vi "MP-Message Decoder.vi"(8 "error in (no error)":errorcluster, 10 "SDO messages":string="#y\u0010\u0000\u0007\u0007\u0001dd\u0001$\u0007\u0007\u0003\u0018ÿ\u0018\u0018\u0018\u0018\u0018\u0018\u0018\u0018)\u0000\u0007\u0007\u0001\u001a", 11 "data controls":T1={"Scan Reset"=FALSE, "Sub Sampling"=1, "Report Data Msg"=FALSE} {"Sub Sampling" items=["", "1:1", "2:1", "3:1", "4:1", "5:1", "6:1", "7:1", "8:1", "9:1", "10:1"]}) -> (0 "error out":errorcluster, 1 "System Status":T5={"System Type"=enum."MicroPulse 5", "Serial No."=0, "Channels"={"Conv"=0, "PA"=0, "Extra"=0}, "Sample Frequency"={"Default"=0, "Actual"=0}, "Software Versions"="", "Data Output Format"={"Default"=enum."8-bit Mode", "Actual"=enum."8-bit Mode"}, "Temperatures"={"System"=0, "Processor"=0, "Slave Sys"=0, "Slave Proc"=0}, "Tx Buffer Size"=0, "System Error"="", "No. of Cards"=0, "DAC Gain"=0, "Uptimes"={"since Power"=0, "since RSTS"=0, "since SRST"=0}, "Voltages"=[], "Interface Cards"=[]} {"Interface Cards"."FPGA - T" format="%.0f °C"; "Interface Cards"."Board - T" format="%.0f °C"; "Voltages"."Difference" format="%.2fV"; "Voltages"."Measured" format="%.2fV"; "Voltages"."Nominal" format="%.2fV"; "DAC Gain" format="%.0fdB"; "Tx Buffer Size" format="%.0fMB"; "Temperatures"."Slave Proc" format="%.0f C"; "Temperatures"."Slave Sys" format="%.0f C"; "Temperatures"."Processor" format="%.0f C"; "Temperatures"."System" format="%.0f C"; "Sample Frequency"."Actual" format="%.0fMHz"; "Sample Frequency"."Default" format="%.0fMHz"}, 2 "scan data info":T9={"Message Header"=0, "Error Message"=0, "Test No."=0, "Channel No."=0, "Sweep No."=0, "Gate No."=0, "DOF"=enum."8-bit Mode", "retain data"=enum."Ascan", "scan data"=[], "scan length"=0, "scan index"=0, "peak data"={"timebase"=[], "data"=[]}, "#peaks"=0, "PRF"=0.0, "IP"={"Axis No."=0, "Location"=0, "MIP location"=0, "MIP?"=FALSE}, "echo range"=0, "ETG"=FALSE, "CAL 0 complete"=FALSE, "Axis Positions"={"Axis 1"=0, "Axis 2"=0, "Axis 3"=0, "Axis 4"=0, "Status"=0}} {"Error Message" format="%04x"; "Message Header" format="%04x"; "IP"."MIP location" format="%#.0f"; "IP"."Location" format="%#.0f"; "PRF" format="%.0fHz"}, 3 "Instrument Message":string="A-Scan\n---------\n\rLength = 108 bytes\nSweep No. 0\nTest No. 0\nDOF = MicroPulse 4\nerror\nChannel No. 0", 4 "reported msg length":u32 format="%d bytes", 5 "Axis Status":T3 {"IO Levels"."Outputs: 7-0" format="%.0b"; "IO Levels"."Outputs: 15-8" format="%.0b"; "IO Levels"."Inputs: 7-0" format="%.0b"; "IO Levels"."Inputs: 15-8" format="%.0b"}, 7 "message header":u16 format="%04x")   [LabVIEW 2026, in "MicroPulse_Driver.lvlib"]
doc: "MicroPulse standard data output message decoder.\n\nNote:\n\n1. Currently only supports LT/LT2 instruments.\n2. Supports LT/LT2/MP5\n3. Supports LTPA.\n\n\nDeon Bester\n2018/11/10"
uses:
  MicroPulse_Driver.lvlib
  Datatypes/MP - scan data info.ctl
  Datatypes/MP - data output format.ctl
  Datatypes/MP - retain scan.ctl
  Datatypes/MP - axis positions (LLC).ctl
  Datatypes/MP - general system status.ctl
  <instrlib>/MicroPulse/Public/Data/Datatypes/MP - instrument type.ctl
  Datatypes/MP - interface card status.ctl
  Datatypes/MP - axis status.ctl
  Datatypes/MP - extracted data controls.ctl
  Datatypes/PNDT - subsampling.ctl
  <vilib>/ptbypt/NI_PtbyPt.lvlib
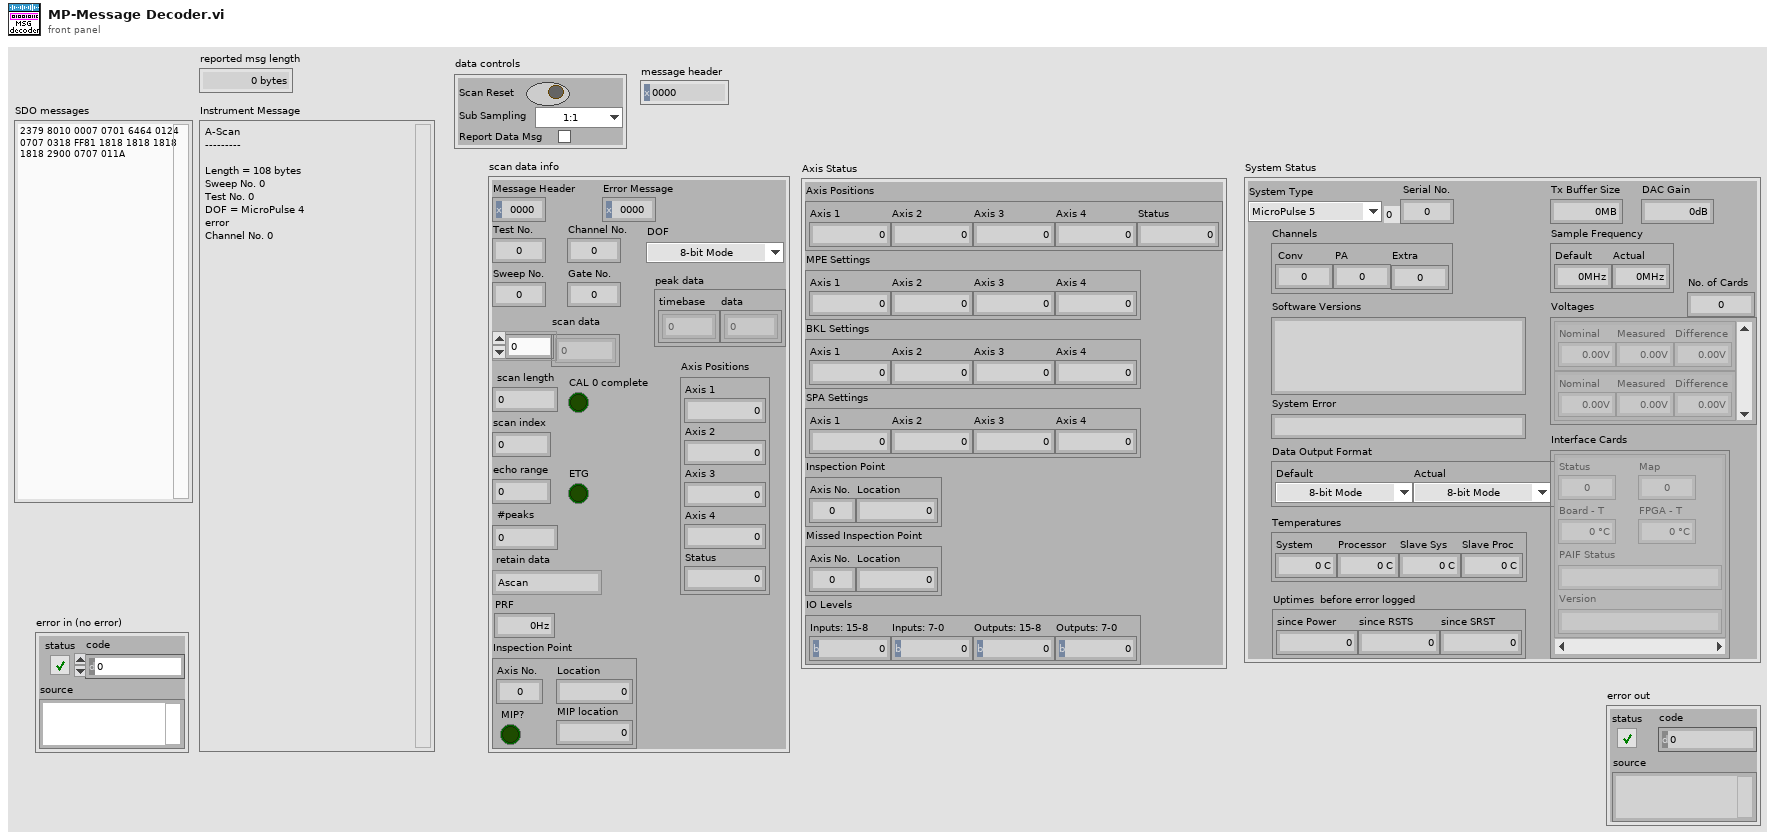
[diagram p1: front panel]
types:
  T1 = typedef "MicroPulse_Driver.lvlib/MP - extracted data controls.ctl" = cluster{"Scan Reset":bool, "Sub Sampling":T2, "Report Data Msg":bool}
  T2 = typedef "MicroPulse_Driver.lvlib/PNDT - subsampling.ctl" = u16
  T3 = typedef "MicroPulse_Driver.lvlib/MP - axis status.ctl" = cluster{"Axis Positions":T4, "MPE Settings":cluster{"Axis 1":u32, "Axis 2":u32, "Axis 3":u32, "Axis 4":u32}, "BKL Settings":cluster{"Axis 1":u32, "Axis 2":u32, "Axis 3":u32, "Axis 4":u32}, "SPA Settings":cluster{"Axis 1":u32, "Axis 2":u32, "Axis 3":u32, "Axis 4":u32}, "IP":cluster{"Axis No.":u8, "Location":u32}, "MIP":cluster{"Axis No.":u8, "Location":u32}, "IO Levels":cluster{"Inputs: 15-8":u8, "Inputs: 7-0":u8, "Outputs: 15-8":u8, "Outputs: 7-0":u8}}
  T4 = typedef "MicroPulse_Driver.lvlib/MP - axis positions (LLC).ctl" = cluster{"Axis 1":u32, "Axis 2":u32, "Axis 3":u32, "Axis 4":u32, "Status":u8}
  T5 = typedef "MicroPulse_Driver.lvlib/MP - general system status.ctl" = cluster{"System Type":T6, "Serial No.":u64, "Channels":cluster{"Conv":u8, "PA":u16, "Extra":u32}, "Sample Frequency":cluster{"Default":u8, "Actual":u8}, "Software Versions":string, "Data Output Format":cluster{"Default":T7, "Actual":T7}, "Temperatures":cluster{"System":u8, "Processor":u8, "Slave Sys":u8, "Slave Proc":u8}, "Tx Buffer Size":u32, "System Error":string, "No. of Cards":u8, "DAC Gain":i16, "Uptimes":cluster{"since Power":u32, "since RSTS":u32, "since SRST":u32}, "Voltages":cluster{"Nominal":dbl, "Measured":dbl, "Difference":dbl}[], "Interface Cards":T8[]}
  T6 = typedef "MicroPulse_Driver.lvlib/MP - instrument type.ctl" = enum16{"MicroPulse 5", "LT1", "LT2", "LTPA", "MPLT", "MicroPulse 6", "PipeScanner", "<MicroPulse>", "Micropulse 4", "Simulated Data"}
  T7 = typedef "MicroPulse_Driver.lvlib/MP - data output format.ctl" = enum16{"", "8-bit Mode", "10-bit Mode", "12-bit Mode", "16-bit Mode", "8-bit Log Mode", "12-bit Packed Mode"}
  T8 = typedef "MicroPulse_Driver.lvlib/MP - interface card status.ctl" = cluster{"Status":u8, "Map":u8, "Board - T":u8, "FPGA - T":u8, "PAIF Status":string, "Version":string}
  T9 = typedef "MicroPulse_Driver.lvlib/MP - scan data info.ctl" = cluster{"Message Header":u16, "Error Message":u16, "Test No.":u32, "Channel No.":u8, "Sweep No.":u32, "Gate No.":u32, "DOF":T7, "retain data":T10, "scan data":u16[], "scan length":i32, "scan index":i32, "peak data":cluster{"timebase":u16[], "data":u16[]}, "#peaks":i32, "PRF":dbl, "IP":cluster{"Axis No.":u8, "Location":u32, "MIP location":u32, "MIP?":bool}, "echo range":u16, "ETG":bool, "CAL 0 complete":bool, "Axis Positions":T4}
  T10 = typedef "MicroPulse_Driver.lvlib/MP - retain scan.ctl" = enum16{"None", "Ascan", "Peaks"}
  T11 = cluster{"Nominal":dbl, "Measured":dbl, "Difference":dbl}[]
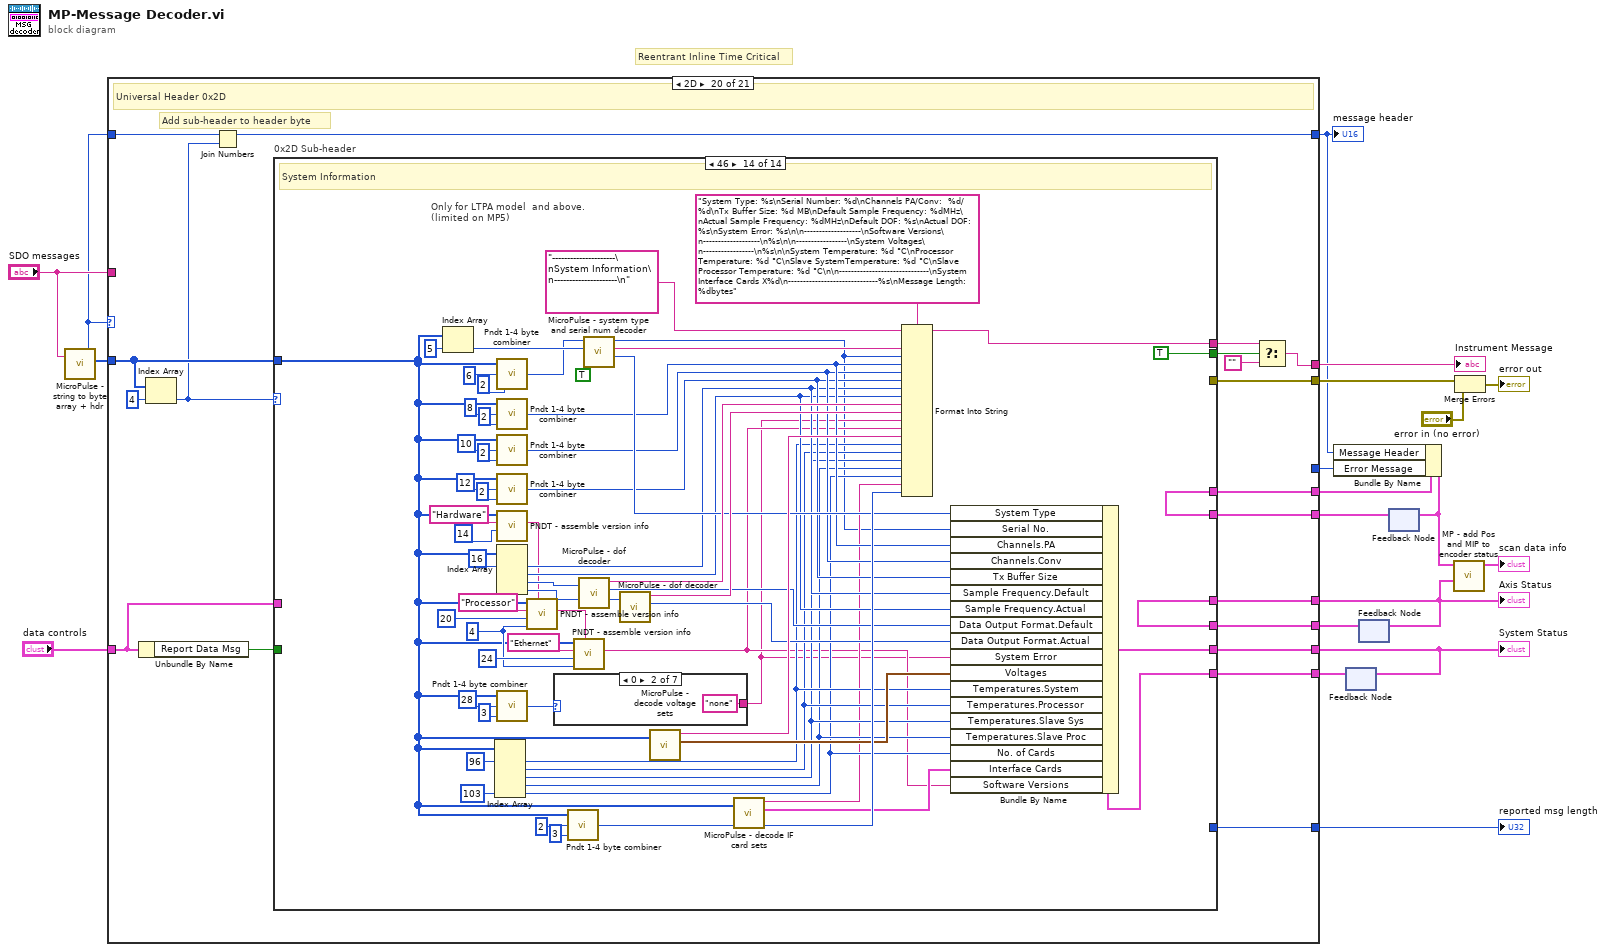
[diagram p0: block diagram]
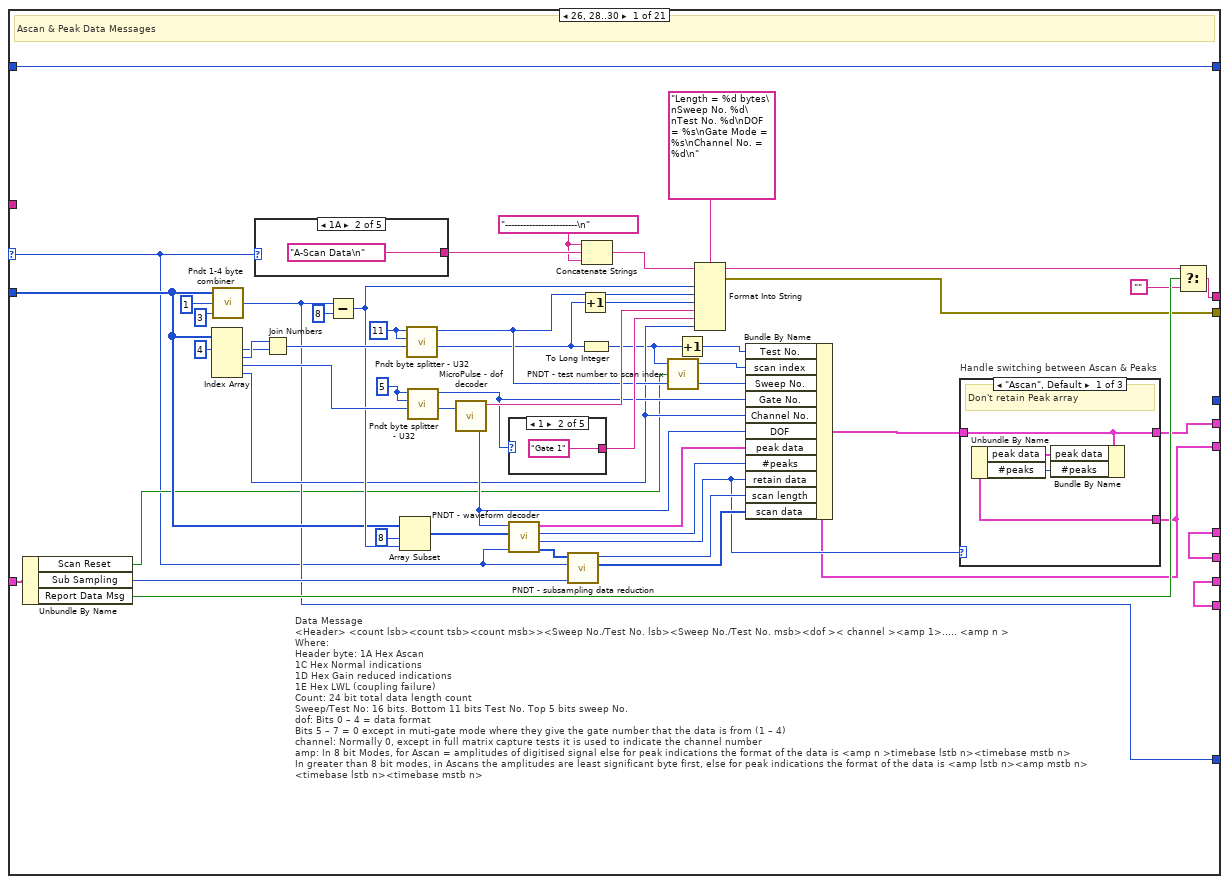
[diagram p2: hidden frame]
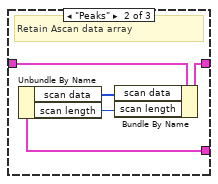
[diagram p3: hidden frame]
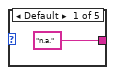
[diagram p5: hidden frame]
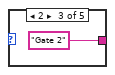
[diagram p6: hidden frame]
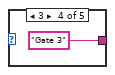
[diagram p7: hidden frame]
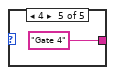
[diagram p8: hidden frame]
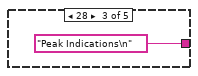
[diagram p10: hidden frame]
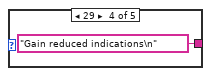
[diagram p11: hidden frame]
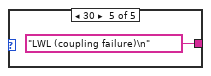
[diagram p12: hidden frame]
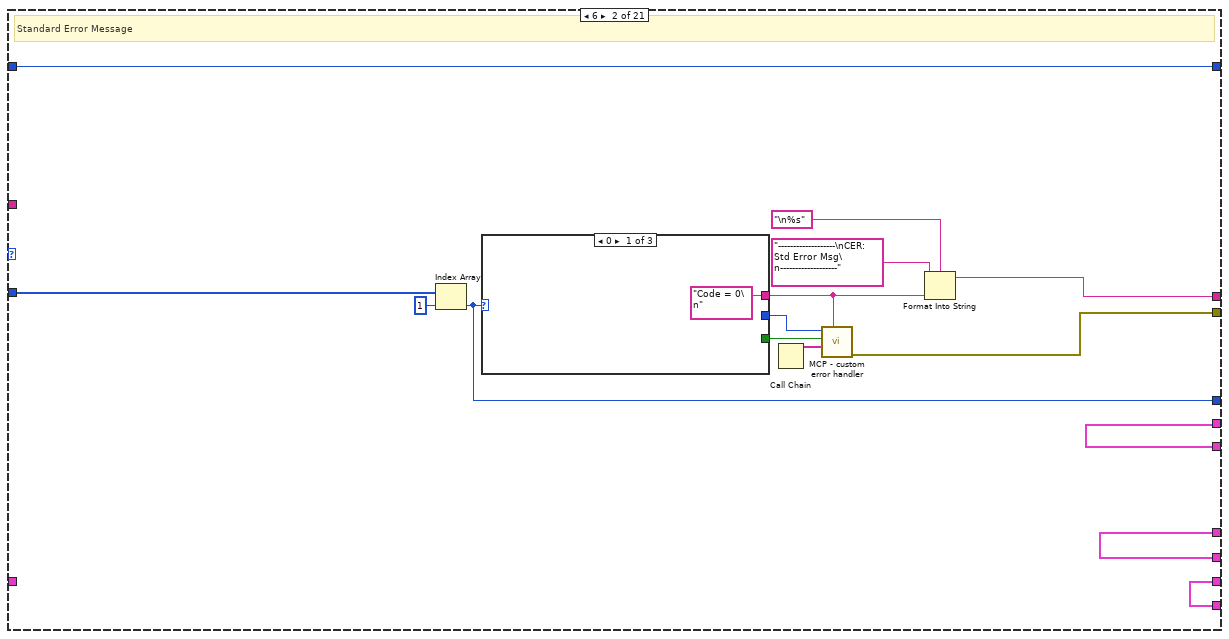
[diagram p13: hidden frame]
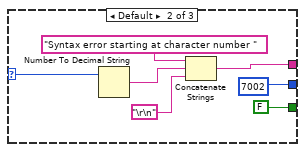
[diagram p14: hidden frame]
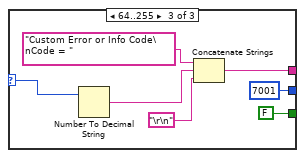
[diagram p15: hidden frame]
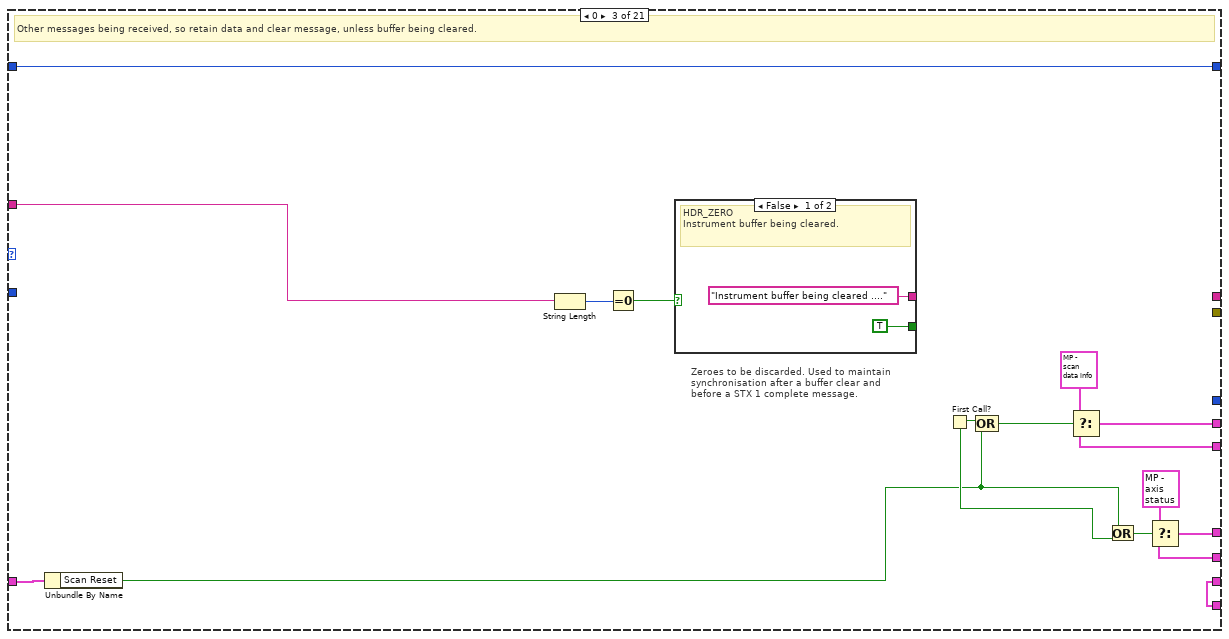
[diagram p16: hidden frame]
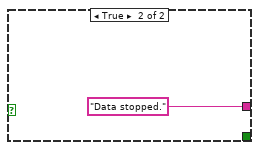
[diagram p17: hidden frame]
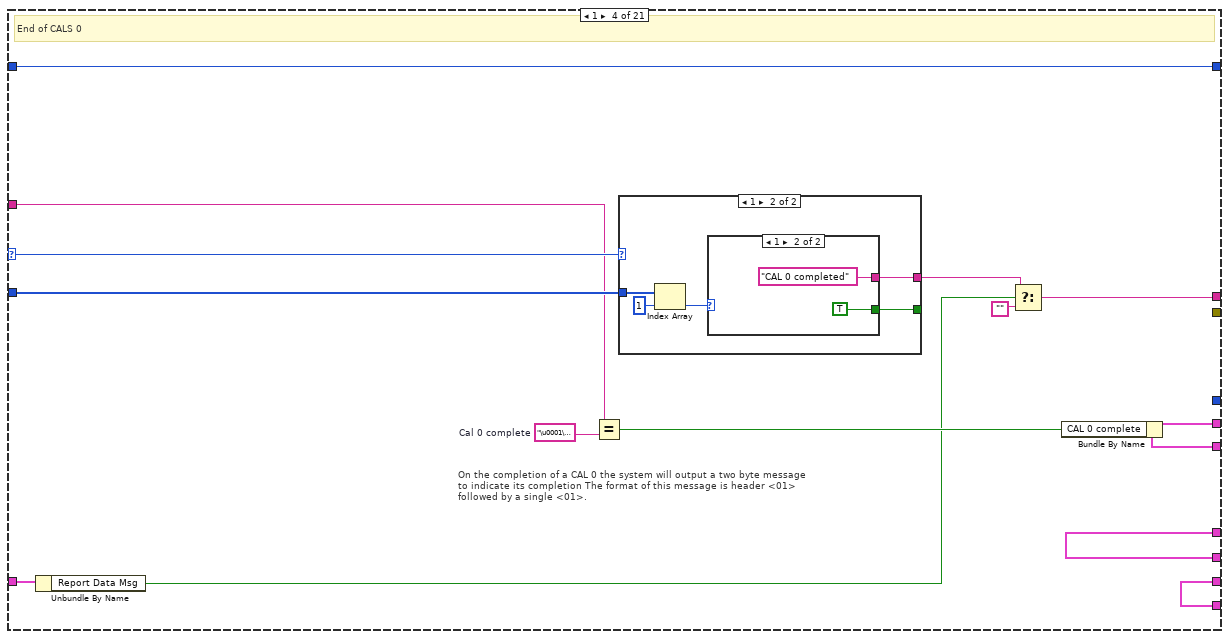
[diagram p18: hidden frame]
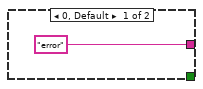
[diagram p19: hidden frame]
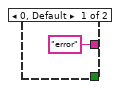
[diagram p20: hidden frame]
diagram:
  # "Reentrant Inline Time Critical"
  n1 = call "MicroPulse - string to byte array + hdr.vi"("SDO msg (hex)"="SDO messages") -> ("header"=w5:u8, "[U8]"=w19:u8[])  [unwired: 3 in]
  n2 = feedback #1() -> (w18:T5)  [unwired: 1 in]
  n3 = feedback #2() -> (w17:T3)  [unwired: 1 in]
  n4 = feedback #3() -> (w14:T9)  [unwired: 1 in]
  n5 = case shown="2D" w5 {
    selector: w5 -> [w24 _ _ w148 _ _ _ _ _ _ _ _ _ _ _ _ _ _ _ _ w1377]
    tunnel: w19 -> [w33 w105 _ w154 w173 w188 w214 w232 w456 w482 w524 w603 w652 w689 w725 w752 w780 w800 w816 w849 _]
    tunnel: [w34 w104 _ w151 w170 w181 w213 w230 w457 w488 w529 w621 w659 w696 w732 w746 w786 w803 w824 w841 w1379] -> w7
    tunnel: w18 -> [w20 w91 w136 w140 w164 w186 w211 w233 w382 w466 w502 _ w631 w668 w705 w741 w770 w790 w807 w847 w1375]
    tunnel: [w28 w99 w129 w152 w166 w175 w210 w231 w384 w468 w504 w574 w633 w670 w707 w748 w772 w792 w809 w845 w1384] -> w16
    tunnel: w17 -> [w28 w99 w130 w152 w166 w187 w212 w235 w384 w468 w504 w574 w633 w670 w707 w748 w772 w792 w809 w846 w1384]
    tunnel: "SDO messages" -> [_ _ w126 w145 _ _ _ _ _ _ _ _ _ _ _ _ _ _ _ _ _]
    tunnel: [w32 w98 _ _ _ _ _ _ _ _ _ _ _ _ _ w751 _ _ _ w844 w1382] -> w6
    tunnel: "data controls" -> [w31 _ w131 w147 _ w180 _ _ _ _ _ _ _ _ _ w745 _ _ _ w838 _]
    tunnel: [w26 w100 w132 w149 w167 w184 w208 w228 w385 w469 w505 w576 w634 w671 w708 w750 w773 w793 w810 w836 w1385] -> w9
    tunnel: w14 -> [w25 w100 w133 w153 w167 w184 w208 w228 w385 w469 w505 w576 w634 w671 w708 w749 w773 w793 w810 w835 w1385]
    tunnel: [w30 _ _ _ _ _ _ _ _ _ _ _ _ _ _ _ _ _ _ w837 _] -> w12
    tunnel: [w21 w93 w121 w141 w165 w179 w206 w227 w383 w467 w503 w573 w632 w669 w706 w743 w771 w791 w808 w833 w1376] -> w3
    tunnel: w5 -> [w21 w93 w121 w141 w165 w179 w206 w227 w383 w467 w503 w573 w632 w669 w706 w743 w771 w791 w808 w834 w1376]
    tunnel: [_ w92 _ _ _ _ _ _ _ _ _ _ _ _ _ _ _ _ _ _ _] -> w2
    tunnel: [w20 w91 w136 w140 w164 w186 w211 w234 w382 w466 w502 w578 w631 w668 w705 w741 w770 w790 w807 w848 w1375] -> w1
    frame 26, 28..30 {
      w64 = i16 11 ("y")
      w66 = i16 5 ("y")
      w49 = "------------------------\n" ("input 1")
      # "Data Message\n<Header> <count lsb><count tsb><count msb>><Sweep No./Test No. lsb><Sweep No./Test No. msb><dof >< channel ><amp 1>….. <amp n >\nWhere:\nHeader byte: 1A Hex Ascan\n1C Hex Normal indications\n1D Hex Gain reduced indications\n1E Hex LWL (coupling failure)\nCount: 24 bit total data length count\nSweep/Test No: 16 bits. Bottom 11 bits Test No. Top 5 bits sweep No.\ndof: Bits 0 – 4 = data format\nBits 5 – 7 = 0 except in muti-gate mode where they give the gate number that the data is from (1 – 4)\nchannel: Normally 0, except in full matrix capture tests it is used to indicate the channel number\namp: In 8 bit Modes, for Ascan = amplitudes of digitised signal else for peak indications the format of the data is <amp n >timebase lstb n><timebase mstb n>\nIn greater than 8 bit modes, in Ascans the amplitudes are least significant byte first, else for peak indications the format of the data is <amp lstb n><amp mstb n> <timebase lstb n><timebase mstb n>"
      # "Ascan & Peak Data Messages"
      n6 = Unbundle By Name(w31) -> ("Scan Reset"=w29:bool, "Sub Sampling"=w46:T2, "Report Data Msg"=w41:bool)
      n7 = Index Array(array=w33, index #1=4 ("index")) -> (element #1=w57:u8, element #2=w58:u8, element #3=w65:u8, element #4=w51:u8)  [unwired: 3 in]
      n8 = call "Pndt 1-4 byte combiner.vi"("#bytes"=3 ("index"), "start index [0]"=1 ("index"), "[U8] count bytes"=w33) -> ("U32"=w30:u32)
      n9 = case shown="1A" w24 {
        tunnel: [_ "A-Scan Data\n" "Peak Indications\n" "Gain reduced indications\n" "LWL (coupling failure)\n"] -> w69
        frame 0, Default {
        }
        frame 26 {
        }
        frame 28 {
        }
        frame 29 {
        }
        frame 30 {
        }
      }
      n10 = Join Numbers(hi=w58, lo=w57) -> ((hi.lo)=w63:u16)
      n11 = Subtract(x=w30, y=u32 8) -> (x-y=w52:u32)
      n12 = Array Subset "Array Subset"(array=w33, index=8, length=w52) -> (w45:u8[])
      n13 = call "Pndt byte splitter - U32.vi"("byte U32"=w63, "mask size"=w64, "shift right"=w64) -> ("lo"=w44:u32, "hi"=w53:u32)  [unwired: 7 in]
      n14 = call "Pndt byte splitter - U32.vi"("byte U32"=w65, "mask size"=w66, "shift right"=w66) -> ("lo"=w61:u32, "hi"=w54:u32)  [unwired: 7 in]
      n15 = call "MicroPulse - dof decoder.vi"("dof"=w61) -> ("String"=w68:string, "DOF"=w55:T7)  [unwired: 3 in]
      n16 = case shown="1" w54 {
        tunnel: ["n.a." "Gate 1" "Gate 2" "Gate 3" "Gate 4"] -> w67
        frame Default {
        }
        frame 1 {
        }
        frame 2 {
        }
        frame 3 {
        }
        frame 4 {
        }
      }
      n17 = call "PNDT - waveform decoder.vi"("header (1A)"=w24, "[U8]"=w45, "DOF"=w55) -> ("scan data"=w48:u16[], "retain data"=w35:T10, "#peaks"=w38:i32, "XY data"=w39:cluster{u16[], u16[]})  [unwired: 5 in]
      n18 = call "PNDT - subsampling data reduction.vi"("sub-sampling"=w46, "header (1A)"=w24, "data set"=w48) -> ("reduced data set"=w40:u16[], "scan length"=w37:i32)  [unwired: 7 in]
      n19 = Increment(x=w44) -> (x+1=w36:u32)
      n20 = To Long Integer(number=w44) -> (32bit integer=w43:i32)
      n21 = Concatenate Strings(w49, w69, w49) -> (w50:string)
      n22 = call "PNDT - test number to scan index.vi"("reset"=w29, "test no."=w43) -> ("scan index"=w42:i32)  [unwired: 2 in, 1 out]
      n23 = Increment(x=w43) -> (x+1=w22:i32)
      n24 = Format Into String(format string="Length = %d bytes\nSweep No. %d\nTest No. %d\nDOF = %s\nGate Mode = %s\nChannel No. = %d\n", initial string=w50, w52, w53, w36, w68, w67, w51) -> (resulting string=w47:string, error out=w32:errorcluster)  [unwired: 1 in]
      n25 = Bundle By Name(cluster=w25, "Test No."=w22, "scan index"=w42, "Sweep No."=w53, "Gate No."=w54, "Channel No."=w51, "DOF"=w55, "peak data"=w39, "#peaks"=w38, "retain data"=w35, "scan length"=w37, "scan data"=w40) -> (w27:T9)
      n26 = case "Handle switching between Ascan & Peaks" shown="\"Ascan\", Default" w35 {
        tunnel: w27 -> [w72 w79 w81]
        tunnel: [w72 w78 w81] -> w26
        tunnel: w25 -> [w74 w77 _]
        frame "Ascan", Default {
          # "Don't retain Peak array"
          n27 = Unbundle By Name(w74) -> ("peak data"=w75:cluster{"timebase":u16[], "data":u16[]}, "#peaks"=w73:i32)
          n28 = Bundle By Name(cluster=w72, "peak data"=w75, "#peaks"=w73) -> ()  [unwired: 1 out]
        }
        frame "Peaks" {
          # "Retain Ascan data array"
          n29 = Unbundle By Name(w77) -> ("scan data"=w80:u16[], "scan length"=w76:i32)
          n30 = Bundle By Name(cluster=w79, "scan data"=w80, "scan length"=w76) -> (w78:T9)
        }
        frame "None" {
        }
      }
      n31 = Select(t=w47, s=w41, f="") -> (s? t:f=w34:string)
    }
    frame 6 {
      # "Standard Error Message"
      n32 = Index Array(array=w105, index=1) -> (element=w92:u8)
      n33 = case shown="0" w92 {
        selector: w92 -> [_ w113 w115]
        tunnel: ["Code = 0\n" w110 w117] -> w95
        tunnel: [_ 7002 ("custom error code") 7001 ("custom error code")] -> w97
        tunnel: [_ FALSE FALSE] -> w94
        frame 0 {
        }
        frame Default {
          n34 = Number To Decimal String(number=w113) -> (decimal integer string=w112:string)  [unwired: 1 in]
          n35 = Concatenate Strings("Syntax error starting at character number " ("input 1"), w112, "\r\n") -> (w110:string)
        }
        frame 64..255 {
          n36 = Number To Decimal String(number=w115) -> (decimal integer string=w118:string)  [unwired: 1 in]
          n37 = Concatenate Strings("Custom Error or Info Code\nCode = " ("input 1"), w118, "\r\n") -> (w117:string)
        }
      }
      n38 = Call Chain() -> (call chain=w96:string[])
      n39 = call "MCP - custom error handler.vi"("message"=w95, "call chain"=w96, "Is Error?"=w94, "custom error code"=w97) -> ("error out"=w98:errorcluster)  [unwired: 7 in]
      n40 = Format Into String(format string="\n%s", initial string="-------------------\nCER: Std Error Msg\n-------------------", w95) -> (resulting string=w104:string)  [unwired: 1 in, 1 out]
    }
    frame 0 {
      # "Zeroes to be discarded. Used to maintain synchronisation after a buffer clear and before a STX 1 complete message."
      # "Other messages being received, so retain data and clear message, unless buffer being cleared."
      n41 = Unbundle By Name(w131) -> ("Scan Reset"=w122:bool)
      n42 = String Length(string=w126) -> (length=w125:i32)
      n43 = Equal To 0?(x=w125) -> (x = 0?=w124:bool)
      n44 = case shown="False" w124 {
        tunnel: ["Instrument buffer being cleared ...." "Data stopped."] -> _
        tunnel: [TRUE _] -> _
        frame False {
          # "HDR_ZERO\nInstrument buffer being cleared."
        }
        frame True {
        }
      }
      n45 = First Call?() -> (First Call?: T/F=w123:bool)
      n46 = Compound Arithmetic op=OR(w123, w122) -> (w135:bool)
      n47 = Select(t=T9 {"Message Header"=0, "Error Message"=0, "Test No."=0, "Channel No."=0, "Sweep No."=0, "Gate No."=0, "DOF"=enum."8-bit Mode", "retain data"=enum."Ascan", "scan data"=[], "scan length"=0, "scan index"=0, "peak data"={"timebase"=[], "data"=[]}, "#peaks"=0, "PRF"=0.0, "IP"={"Axis No."=0, "Location"=0, "MIP location"=0, "MIP?"=FALSE}, "echo range"=0, "ETG"=FALSE, "CAL 0 complete"=FALSE, "Axis Positions"={"Axis 1"=0, "Axis 2"=0, "Axis 3"=0, "Axis 4"=0, "Status"=0}}, s=w135, f=w133) -> (s? t:f=w132:T9)
      n48 = Or(x=w122, y=w123) -> (x .or. y?=w128:bool)
      n49 = Select(t=T3 {"Axis Positions"={"Axis 1"=0, "Axis 2"=0, "Axis 3"=0, "Axis 4"=0, "Status"=0}, "MPE Settings"={"Axis 1"=0, "Axis 2"=0, "Axis 3"=0, "Axis 4"=0}, "BKL Settings"={"Axis 1"=0, "Axis 2"=0, "Axis 3"=0, "Axis 4"=0}, "SPA Settings"={"Axis 1"=0, "Axis 2"=0, "Axis 3"=0, "Axis 4"=0}, "IP"={"Axis No."=0, "Location"=0}, "MIP"={"Axis No."=0, "Location"=0}, "IO Levels"={"Inputs: 15-8"=0, "Inputs: 7-0"=0, "Outputs: 15-8"=0, "Outputs: 7-0"=0}}, s=w128, f=w130) -> (s? t:f=w129:T3)
    }
    frame 1 {
      w146 = "\u0001\u0001"  # Cal 0 complete
      # "On the completion of a CAL 0 the system will output a two byte message to indicate its completion The format of this message is header <01> followed by a single <01>."
      # "End of CALS 0"
      n50 = Unbundle By Name(w147) -> ("Report Data Msg"=w142:bool)
      n51 = Equal?(x=w145, y=w146) -> (x = y?=w144:bool)
      n52 = case shown="1" w148 {
        tunnel: ["error" w157] -> w143
        tunnel: w154 -> [_ w160]
        tunnel: [_ w156] -> _
        frame 0, Default {
        }
        frame 1 {
          n53 = Index Array(array=w160, index=1) -> (element=w159:u8)
          n54 = case shown="1" w159 {
            tunnel: ["error" ("input 1") "CAL 0 completed" ("input 1")] -> w157
            tunnel: [_ TRUE] -> w156
            frame 0, Default {
            }
            frame 1 {
            }
          }
        }
      }
      n55 = Select(t=w143, s=w142, f="") -> (s? t:f=w151:string)
      n56 = Bundle By Name(cluster=w153, "CAL 0 complete"=w144) -> (w149:T9)
    }
    frame 8 {
      # "If no signal appears in the echo gate above the EUPL then a two byte ING message is reported: $8<Tn>"
      # "ING - Interface echo trigger failure"
      n57 = Index Array(array=w173, index=1) -> (element=w168:u8)
      n58 = Format Into String(format string="Test No. %d", initial string="\n-----------------\nING: Interface echo trigger failure\n-----------------", w168) -> (resulting string=w170:string)  [unwired: 1 in, 1 out]
    }
    frame 19 {
      # "copy location into LLC record"
      # "LCI message\nThe LCI message is output during a moving inspection mode. It precedes any data from an inspection point and gives the actual location of that inspection point.\n(24 Bit mode)\n<Header 0x13><axis><K axis>\nWhere:\naxis: Axis number n\nKn: Three byte location of axis n, least significant first."
      # "LCI  - Inspection Point Location"
      n59 = Unbundle By Name(w180) -> ()  [unwired: 1 out]
      n60 = Index Array(array=w188, index=1) -> (element=w178:u8)
      n61 = call "Pndt 1-4 byte combiner.vi"("#bytes"=3, "start index [0]"=2, "[U8] count bytes"=w188) -> ("U32"=w177:u32)
      n62 = Format Into String(format string="\nAxis No. %d\nInspection Point Location: %d", initial string="--------------------\nLCI MESSAGE (24b)\n--------------------", w178, w177) -> (resulting string=w182:string)  [unwired: 1 in, 1 out]
      n63 = Bundle By Name(cluster=w187, "IP.Axis No."=w178, "IP.Location"=w177) -> (w176:T3)
      n64 = case shown="4" w178 {
        tunnel: w176 -> [w193 w196 w199 w202 w205]
        tunnel: [w193 w195 w198 w201 w204] -> w175
        tunnel: w177 -> [_ w194 w197 w200 w203]
        frame 0, Default {
          # "Error - Do nothing"
        }
        frame 1 {
          n65 = Bundle By Name(cluster=w196, "Axis Positions.Axis 1"=w194) -> (w195:T3)
        }
        frame 2 {
          n66 = Bundle By Name(cluster=w199, "Axis Positions.Axis 2"=w197) -> (w198:T3)
        }
        frame 3 {
          n67 = Bundle By Name(cluster=w202, "Axis Positions.Axis 3"=w200) -> (w201:T3)
        }
        frame 4 {
          n68 = Bundle By Name(cluster=w205, "Axis Positions.Axis 4"=w203) -> (w204:T3)
        }
      }
      n69 = Select(t=w182, s=TRUE, f="") -> (s? t:f=w181:string)
    }
    frame 20 {
      # "LCA message\nThe LCA message is used to indicate a missed inspection point. The format of this message is as shown above, unless the message is generated due to the MicroPulse buffer being full. In this case the LCA has the top bit of the axis byte is set to 1.\n(24 Bit mode)\n<Header 0x14><axis><K axis>\nWhere:\nStatus: Status Byte\nKn: Three byte location of axis n, least significant first."
      # "LCA  - Missed Inspection Point"
      n70 = call "Pndt 1-4 byte combiner.vi"("#bytes"=3, "start index [0]"=2, "[U8] count bytes"=w214) -> ("U32"=w223:u32)
      n71 = Index Array(array=w214, index=1) -> (element=w221:u8)
      n72 = call "Pndt byte splitter - U32.vi"("byte U32"=w221, "shift right"=i16 7) -> ("hi"=w218:u32)  [unwired: 8 in, 1 out]
      n73 = case shown="0, Default" w218 {
        tunnel: w221 -> [w225 _]
        tunnel: [w225 _] -> w207
        tunnel: [w224 "Error: Buffer FULL"] -> w222
        frame 0, Default {
          n74 = Format Into String(w225) -> (resulting string=w224:string)  [unwired: 3 in, 1 out]
        }
        frame 1 {
        }
      }
      n75 = Format Into String(format string="\nAxis No. %s\nMissed Inspection Point:  %d", initial string="---------------------\nLCA MESSAGE (24b)\n---------------------", w222, w223) -> (resulting string=w213:string)  [unwired: 1 in, 1 out]
      n76 = Bundle By Name(cluster=w212, "MIP.Axis No."=w207, "MIP.Location"=w223) -> (w210:T3)
    }
    frame 21 {
      # "LLC message\nThe LLC message is generated in response to a STAor STS 0 command and gives the current location for all axes.\n(24 Bit mode)\n<Header 0x15><status>< K1><K2><K3><K4><Info>\nWhere:\nStatus: Status Byte (reflection of the optional parameter in STA)\nKn: Three byte location of axis n, least significant first.\nInfo: Four Bytes normally set to 0xffffffff, but in moving inspection modes can be configured to give information on the number of Bytes left in the system buffer when the test was fired (Status = 1)."
      # "LLC (24b)  - axis and system status"
      n77 = Index Array(array=w232, index=1) -> (element=w237:u8)
      n78 = case shown="F7" w237 {
        selector: w237 -> [_ w242 w271 w289 w317 w324 w348 w367 w378]
        tunnel: w232 -> [_ w246 w278 w296 w315 w331 w346 w358 w374]
        tunnel: [w238 w253 w273 w291 w309 w326 w350 w366 w380] -> w231
        tunnel: [_ w252 w272 w290 w318 w325 w349 w368 w371] -> w230
        tunnel: w235 -> [w240 w250 w269 w286 w309 w322 w340 w366 w380]
        tunnel: w233 -> [w241 w249 w268 w287 w308 w321 w339 w357 w381]
        tunnel: [w241 w249 w268 w287 w307 w321 w339 w356 w381] -> w234
        tunnel: "--------------------\nLLC MESSAGE (24b)\n--------------------\n" -> [_ w243 w267 w285 w303 w320 w338 w352 w370]
        frame Default {
          n79 = Variant To Data(type=T3 {"Axis Positions"={"Axis 1"=0, "Axis 2"=0, "Axis 3"=0, "Axis 4"=0, "Status"=0}, "MPE Settings"={"Axis 1"=0, "Axis 2"=0, "Axis 3"=0, "Axis 4"=0}, "BKL Settings"={"Axis 1"=0, "Axis 2"=0, "Axis 3"=0, "Axis 4"=0}, "SPA Settings"={"Axis 1"=0, "Axis 2"=0, "Axis 3"=0, "Axis 4"=0}, "IP"={"Axis No."=0, "Location"=0}, "MIP"={"Axis No."=0, "Location"=0}, "IO Levels"={"Inputs: 15-8"=0, "Inputs: 7-0"=0, "Outputs: 15-8"=0, "Outputs: 7-0"=0}} ("Axis Status"), Variant=w240) -> (data=w238:T3)  [unwired: 1 in, 1 out]
        }
        frame 0, 1, 240 {
          w258 = 3 ("#bytes")
          # "STA/STS 0 - Axis Locations"
          n80 = call "Pndt 1-4 byte combiner.vi"("#bytes"=4, "start index [0]"=14, "[U8] count bytes"=w246) -> ("U32"=w244:u32)
          n81 = call "Pndt 1-4 byte combiner.vi"("#bytes"=w258, "start index [0]"=2, "[U8] count bytes"=w246) -> ("U32"=w257:u32)
          n82 = call "Pndt 1-4 byte combiner.vi"("#bytes"=w258, "start index [0]"=5, "[U8] count bytes"=w246) -> ("U32"=w256:u32)
          n83 = call "Pndt 1-4 byte combiner.vi"("#bytes"=w258, "start index [0]"=8, "[U8] count bytes"=w246) -> ("U32"=w255:u32)
          n84 = call "Pndt 1-4 byte combiner.vi"("#bytes"=w258, "start index [0]"=11, "[U8] count bytes"=w246) -> ("U32"=w254:u32)
          n85 = case shown="Default" w244 {
            tunnel: [w265 _] -> w245
            tunnel: w244 -> [w264 _]
            frame Default {
              n86 = Format Into String(format string="Bytes left in Buffer = %d", w264) -> (resulting string=w265:string)  [unwired: 2 in, 1 out]
            }
            frame 0, -1 {
            }
          }
          n87 = Format Into String(format string="\nStatus %x\n%s\nAxis 1: %d\nAxis 2: %d\nAxis 3: %d\nAxis 4: %d\n%s", initial string=w243, w242, "Axis Locations", w257, w256, w255, w254, w245) -> (resulting string=w252:string)  [unwired: 1 in, 1 out]
          n88 = Bundle By Name(cluster=w250, "Axis Positions.Status"=w242, "Axis Positions.Axis 1"=w257, "Axis Positions.Axis 2"=w256, "Axis Positions.Axis 3"=w255, "Axis Positions.Axis 4"=w254) -> (w253:T3)
        }
        frame 241 {
          w279 = 3 ("#bytes")
          # "STS 1 - MPE Settings"
          n89 = call "Pndt 1-4 byte combiner.vi"("#bytes"=w279, "start index [0]"=2, "[U8] count bytes"=w278) -> ("U32"=w277:u32)
          n90 = call "Pndt 1-4 byte combiner.vi"("#bytes"=w279, "start index [0]"=5, "[U8] count bytes"=w278) -> ("U32"=w276:u32)
          n91 = call "Pndt 1-4 byte combiner.vi"("#bytes"=w279, "start index [0]"=8, "[U8] count bytes"=w278) -> ("U32"=w275:u32)
          n92 = call "Pndt 1-4 byte combiner.vi"("#bytes"=w279, "start index [0]"=11, "[U8] count bytes"=w278) -> ("U32"=w274:u32)
          n93 = Format Into String(format string="\nStatus %x\n%s\nAxis 1: %d\nAxis 2: %d\nAxis 3: %d\nAxis 4 %d", initial string=w267, w271, "MPE Settings", w277, w276, w275, w274) -> (resulting string=w272:string)  [unwired: 1 in, 1 out]
          n94 = Bundle By Name(cluster=w269, "MPE Settings.Axis 1"=w277, "MPE Settings.Axis 2"=w276, "MPE Settings.Axis 3"=w275, "MPE Settings.Axis 4"=w274) -> (w273:T3)
        }
        frame 242 {
          w297 = 3 ("#bytes")
          # "STS 2 - BKL Settings"
          n95 = call "Pndt 1-4 byte combiner.vi"("#bytes"=w297, "start index [0]"=2, "[U8] count bytes"=w296) -> ("U32"=w295:u32)
          n96 = call "Pndt 1-4 byte combiner.vi"("#bytes"=w297, "start index [0]"=5, "[U8] count bytes"=w296) -> ("U32"=w294:u32)
          n97 = call "Pndt 1-4 byte combiner.vi"("#bytes"=w297, "start index [0]"=8, "[U8] count bytes"=w296) -> ("U32"=w293:u32)
          n98 = call "Pndt 1-4 byte combiner.vi"("#bytes"=w297, "start index [0]"=11, "[U8] count bytes"=w296) -> ("U32"=w292:u32)
          n99 = Format Into String(format string="\nStatus %x\n%s\nAxis 1: %d\nAxis 2: %d\nAxis 3: %d\nAxis 4 %d", initial string=w285, w289, "BKL Settings", w295, w294, w293, w292) -> (resulting string=w290:string)  [unwired: 1 in, 1 out]
          n100 = Bundle By Name(cluster=w286, "BKL Settings.Axis 1"=w295, "BKL Settings.Axis 1"=w294, "BKL Settings.Axis 3"=w293, "BKL Settings.Axis 4"=w292) -> (w291:T3)
        }
        frame 244 {
          # "STS 20 - System Temperatures"
          n101 = Index Array(array=w315, index #1=2 ("index"), index #2=4 ("index"), index #3=6 ("index"), index #4=8 ("index")) -> (element #1=w313:u8, element #2=w312:u8, element #3=w311:u8, element #4=w310:u8)
          n102 = Format Into String(format string="Status %x\n\n%s\nSystem %d degC\nPocessor %d degC\nSlave System %d degC\nSlave Processor %d degC", initial string=w303, w317, "---------------------------\nInstrument Temperatures\n---------------------------", w313, w312, w311, w310) -> (resulting string=w318:string)  [unwired: 1 in, 1 out]
          n103 = Bundle By Name(cluster=w308, "Temperatures.System"=w313, "Temperatures.Processor"=w312, "Temperatures.Slave Sys"=w311, "Temperatures.Slave Proc"=w310) -> (w307:T5)
        }
        frame 245 {
          w332 = 3 ("#bytes")
          # "STS 5 - SPA Settings"
          n104 = call "Pndt 1-4 byte combiner.vi"("#bytes"=w332, "start index [0]"=2, "[U8] count bytes"=w331) -> ("U32"=w330:u32)
          n105 = call "Pndt 1-4 byte combiner.vi"("#bytes"=w332, "start index [0]"=5, "[U8] count bytes"=w331) -> ("U32"=w329:u32)
          n106 = call "Pndt 1-4 byte combiner.vi"("#bytes"=w332, "start index [0]"=8, "[U8] count bytes"=w331) -> ("U32"=w328:u32)
          n107 = call "Pndt 1-4 byte combiner.vi"("#bytes"=w332, "start index [0]"=11, "[U8] count bytes"=w331) -> ("U32"=w327:u32)
          n108 = Format Into String(format string="\nStatus %x\n%s\nAxis 1: %d\nAxis 2: %d\nAxis 3: %d\nAxis 4 %d", initial string=w320, w324, "SPA Settings", w330, w329, w328, w327) -> (resulting string=w325:string)  [unwired: 1 in, 1 out]
          n109 = Bundle By Name(cluster=w322, "SPA Settings.Axis 1"=w330, "SPA Settings.Axis 2"=w329, "SPA Settings.Axis 3"=w328, "SPA Settings.Axis 4"=w327) -> (w326:T3)
        }
        frame 246 {
          # "STS 6 - I/O Line Status"
          n110 = Index Array(array=w346, index #1=2 ("index")) -> (element #1=w344:u8, element #2=w343:u8, element #3=w342:u8, element #4=w341:u8)  [unwired: 4 in, 1 out]
          n111 = Format Into String(format string="\nStatus %x\n%s\nInputs 15-8: %08b\nInputs 7-0: %08b\nOutputs 15-8: %08b\nOutputs 7-0: %08b", initial string=w338, w348, "I/O Status", w344, w343, w342, w341) -> (resulting string=w349:string)  [unwired: 1 in, 1 out]
          n112 = Bundle By Name(cluster=w340, "IO Levels.Inputs: 15-8"=w344, "IO Levels.Inputs: 7-0"=w343, "IO Levels.Outputs: 15-8"=w342, "IO Levels.Outputs: 7-0"=w341) -> (w350:T3)
        }
        frame 247 {
          # "STS 7 - Uptimes since last reset"
          n113 = call "Pndt 1-4 byte combiner.vi"("#bytes"=4 ("index"), "start index [0]"=12 ("index"), "[U8] count bytes"=w358) -> ("U32"=w353:u32)
          n114 = call "Pndt 1-4 byte combiner.vi"("#bytes"=4 ("index"), "start index [0]"=4 ("index"), "[U8] count bytes"=w358) -> ("U32"=w355:u32)
          n115 = call "Pndt 1-4 byte combiner.vi"("#bytes"=4 ("index"), "start index [0]"=8 ("index"), "[U8] count bytes"=w358) -> ("U32"=w354:u32)
          n116 = call "MicroPulse - uptime msg assembly.vi"("SRST"=w353, "RST"=w354, "Uptime"=w355) -> ("String"=w359:string)  [unwired: 8 in]
          n117 = Format Into String(format string="\nStatus %x\n%s", initial string=w352, w367, w359) -> (resulting string=w368:string)  [unwired: 1 in, 1 out]
          n118 = Bundle By Name(cluster=w357, "Uptimes.since Power"=w355, "Uptimes.since RSTS"=w354, "Uptimes.since SRST"=w353) -> (w356:T5)
        }
        frame 248 {
          # "STS 8 - System Information"
          n119 = Array Subset(array=w374, index=2) -> (w372:u8[])  [unwired: 1 in]
          n120 = Number To Hexadecimal String(1:u8 2 ("width (-)"), 2:w372) -> (0:w377:string[])
          n121 = Concatenate Strings(w377) -> (w376:string)
          n122 = Format Into String(format string="\nStatus %x\nSys Info %s", initial string=w370, w378, w376) -> (resulting string=w371:string)  [unwired: 1 in, 1 out]
        }
      }
    }
    frame 32 {
      w453 = i16 4 ("shift right")
      # "Spare"
      # "XXA response message"
      n123 = Index Array(array=w456, index #1=1 ("index"), index #25=24 ("index")) -> (element #1=w393:u8, element #2=w392:u8, element #3=w394:u8, element #4=w395:u8, element #5=w396:u8, element #6=w397:u8, element #7=w398:u8, element #8=w399:u8, element #9=w400:u8, element #10=w401:u8, element #11=w402:u8, element #12=w449:u8, element #13=w450:u8, element #14=w448:u8, element #15=w447:u8, element #16=w444:u8, element #17=w443:u8, element #18=w441:u8, element #19=w440:u8, element #20=w437:u8, element #21=w438:u8, element #22=w436:u8, element #23=w435:u8, element #25=w427:u8, element #26=w426:u8, element #27=w423:u8, element #28=w424:u8, element #29=w421:u8, element #30=w420:u8, element #31=w414:u8, element #32=w413:u8, element #33=w412:u8, element #34=w411:u8, element #35=w409:u8, element #36=w408:u8, element #37=w405:u8, element #38=w406:u8, element #39=w403:u8, element #40=w404:u8)  [unwired: 38 in, 1 out]
      n124 = Join Numbers(hi=w404, lo=w403) -> ()  [unwired: 1 out]
      n125 = Join Numbers(hi=w411, lo=w412) -> ((hi.lo)=w410:u16)
      n126 = Join Numbers(hi=w408, lo=w409) -> ((hi.lo)=w407:u16)
      n127 = Join Numbers(hi=w406, lo=w405) -> ((hi.lo)=w388:u16)
      n128 = Join Numbers(hi=w392, lo=w393) -> ((hi.lo)=w389:u16)
      n129 = Join Numbers(hi=w395, lo=w394) -> ((hi.lo)=w455:u16)
      n130 = Join Numbers(hi=w397, lo=w396) -> ((hi.lo)=w454:u16)
      n131 = Join Numbers(hi=w450, lo=w449) -> ((hi.lo)=w446:u16)
      n132 = Join Numbers(hi=w447, lo=w448) -> ((hi.lo)=w445:u16)
      n133 = Join Numbers(hi=w443, lo=w444) -> ((hi.lo)=w442:u16)
      n134 = Join Numbers(hi=w440, lo=w441) -> ((hi.lo)=w439:u16)
      n135 = Join Numbers(hi=w438, lo=w437) -> ((hi.lo)=w434:u16)
      n136 = Join Numbers(hi=w435, lo=w436) -> ((hi.lo)=w428:u16)
      n137 = Join Numbers(hi=w426, lo=w427) -> ((hi.lo)=w425:u16)
      n138 = Join Numbers(hi=w424, lo=w423) -> ((hi.lo)=w422:u16)
      n139 = Number To Boolean Array(number=w420) -> (Boolean array=w433:bool[])
      n140 = call "MicroPulse - decode amp-reporting mode.vi"("Byte0"=w402, "Byte 1"=w401, "Byte 2"=w400, "Byte 3"=w399) -> ("script"=w390:string)
      n141 = Index Array(array=w433, index #1=7 ("index"), index #2=6 ("index"), index #3=5 ("index")) -> (element #1=w429:bool, element #2=w419:bool, element #3=w416:bool)
      n142 = call "Pndt byte splitter - U32.vi"("byte U32"=w398, "mask size"=w453, "shift right"=w453) -> ("lo"=w451:u32, "hi"=w452:u32)  [unwired: 7 in]
      n143 = case shown="False" w429 {
        tunnel: ["Test ON" "Test OFF"] -> w418
        frame True {
        }
        frame False {
        }
      }
      n144 = case shown="False" w416 {
        tunnel: ["Interface Echo" "Initial Pulse"] -> w415
        frame True {
        }
        frame False {
        }
      }
      n145 = Increment(x=w388) -> (x+1=w387:u16)
      n146 = case shown="True" w419 {
        tunnel: ["DAC ON" "DAC OFF"] -> w417
        frame True {
        }
        frame False {
        }
      }
      n147 = Format Into String(format string="\nTest No. %d\nTx Focal Law %d\nRx Focal Law (Chan No) %d\nGain: %ddB\nFilter: %d\nSmoothing: %d\n%s\nGate Start/End: %d - %d\nDelay = %d\nIG trigger level - UML = %d\n\nEcho Gate Mode\n------------------\nEcho Gate Start/End:   %d - %d\nInspection Gate Start/End:   %d - %d\n\nHysteresis: %d\n%s\n%s\nEcho Trigger Mode: %s\nDAC No. %d\nTest  Sample Frequency = %d\nVelocity for this test: %d\nEG trigger level (EUPL) = %d", initial string="---------------\nXXA Response\n---------------", w389, w455, w387, w454, w451, w452, w390, w446, w445, w442, w439, w434, w428, w425, w422, w421, w418, w417, w415, w414, w413, w410, w407) -> (resulting string=w457:string)  [unwired: 1 in, 1 out]
    }
    frame 33 {
      # "XXAS - Sweep No."
      n148 = Index Array(array=w482, index #1=1 ("index")) -> (element #1=w486:u8, element #2=w485:u8, element #3=w475:u8, element #4=w473:u8, element #5=w474:u8, element #6=w471:u8, element #7=w470:u8)  [unwired: 6 in]
      n149 = Array Subset(array=w482, index=8) -> (w480:u8[])  [unwired: 1 in]
      n150 = Join Numbers(hi=w470, lo=w471) -> ((hi.lo)=w483:u16)
      n151 = Join Numbers(hi=w485, lo=w486) -> ((hi.lo)=w487:u16)
      n152 = To Long Integer(number=w483) -> (32bit integer=w476:i32)
      n153 = for {
        N: w476 -> [_]
        tunnel: w480 -> [w501]
        tunnel: [w493] -> w479 mode=indexing
        i -> [w499]
        w498 = 2 ("x")
        n154 = Multiply(x=w499, y=w498) -> (x*y=w500:i32)
        n155 = Array Subset(array=w501, index=w500, length=w498) -> (w497:u8[])
        n156 = Index Array(array=w497) -> (element #1=w496:u8, element #2=w494:u8)  [unwired: 2 in]
        n157 = Join Numbers(hi=w494, lo=w496) -> ()  [unwired: 1 out]
        n158 = Format Into String(format string="%d ", w494) -> (resulting string=w493:string)  [unwired: 2 in, 1 out]
      }
      n159 = case shown="0" w473 {
        tunnel: ["Enabled" ("format string") "Disabled" ("format string") _] -> w472
        frame 1 {
        }
        frame 0 {
        }
        frame Default {
        }
      }
      n160 = Concatenate Strings("Test Numbers = " ("format string"), w479) -> (w478:string)
      n161 = Format Into String(format string="\nMessage Count %d\nSweep No. %d\nSweep State = %s\nSpare = %d\nNo. of Tests in Sweep = %d\n%s\n", initial string="----------------\nXXAS Response\n----------------", w487, w475, w472, w474, w483, w478) -> (resulting string=w488:string)  [unwired: 1 in, 1 out]
    }
    frame 34 {
      # "XXT/XXR - Tx/Rx Focal Law No."
      n162 = Index Array(array=w524, index #1=1 ("index")) -> (element #1=w527:u8, element #2=w526:u8, element #3=w506:u8, element #4=w515:u8, element #5=w516:u8, element #6=w519:u8, element #7=w518:u8)  [unwired: 6 in]
      n163 = Array Subset(array=w524, index=8, length=520) -> (w522:u8[])
      n164 = Join Numbers(hi=w526, lo=w527) -> ((hi.lo)=w528:u16)
      n165 = Join Numbers(hi=w516, lo=w515) -> ((hi.lo)=w514:u16)
      n166 = Join Numbers(hi=w518, lo=w519) -> ((hi.lo)=w513:u16)
      n167 = case shown="0" w506 {
        tunnel: ["gain trim =%d\n" ("format string") "volatge apod =%d\n" ("format string") _] -> w507
        frame 0 {
        }
        frame 1 {
        }
        frame Default {
        }
      }
      n168 = case shown="1" w506 {
        tunnel: ["Tx Focal Law" ("format string") "Rx Focal Law" ("format string") _] -> w517
        frame 1 {
        }
        frame 0 {
        }
        frame Default {
        }
      }
      n169 = Concatenate Strings("Chan %d: delay =%d  " ("format string"), w507) -> (w508:string)
      n170 = for {
        N: 128 -> [_]
        tunnel: w522 -> [w549]
        tunnel: [w543] -> w521 mode=indexing
        tunnel: w508 -> [w540]
        i -> [w542]
        w547 = 4 ("x")
        n171 = Multiply(x=w542, y=w547) -> (x*y=w548:i32)
        n172 = Array Subset(array=w549, index=w548, length=w547) -> (w546:u8[])
        n173 = Index Array(array=w546) -> (element #1=w545:u8, element #2=w544:u8, element #3=w538:u8, element #4=w537:u8)  [unwired: 4 in]
        n174 = Increment(x=w542) -> (x+1=w541:i32)
        n175 = Join Numbers(hi=w544, lo=w545) -> ((hi.lo)=w539:u16)
        n176 = Join Numbers(hi=w537, lo=w538) -> ((hi.lo)=w536:u16)
        n177 = Format Into String(format string=w540, w541, w539, w536) -> (resulting string=w543:string)  [unwired: 2 in, 1 out]
      }
      n178 = Concatenate Strings("Focal Law Channels\n--------------------\n " ("format string"), w521) -> (w510:string)
      n179 = Format Into String(format string="\nMessage Count %d\n%s\nFocal Law No. %d\nSpare = %d\n%s\n", initial string="--------------------\nXXT/XXR Response\n--------------------", w528, w517, w514, w513, w510) -> (resulting string=w529:string)  [unwired: 1 in, 1 out]
    }
    frame 35 {
      w564 = T5 {"System Type"=enum."MicroPulse 5", "Serial No."=0, "Channels"={"Conv"=0, "PA"=0, "Extra"=0}, "Sample Frequency"={"Default"=0, "Actual"=0}, "Software Versions"="", "Data Output Format"={"Default"=enum."8-bit Mode", "Actual"=enum."8-bit Mode"}, "Temperatures"={"System"=0, "Processor"=0, "Slave Sys"=0, "Slave Proc"=0}, "Tx Buffer Size"=0, "System Error"="", "No. of Cards"=0, "DAC Gain"=0, "Uptimes"={"since Power"=0, "since RSTS"=0, "since SRST"=0}, "Voltages"=[], "Interface Cards"=[]}  # system status
      w611 = i16 5 ("y")
      # "RST Status Message"
      n180 = Index Array(array=w603, index #1=7 ("index")) -> (element #1=w602:u8, element #2=w583:u8, element #3=w582:u8, element #4=w600:u8, element #5=w604:u8)  [unwired: 4 in]
      n181 = Index Array(array=w603, index #1=1 ("index"), index #2=4 ("index")) -> (element #1=w599:u8, element #2=w567:u8)
      n182 = Index Array(array=w603, index #1=17 ("index"), index #2=2 ("index")) -> (element #1=w565:u8, element #2=w612:u8, element #3=w571:u8)  [unwired: 1 in]
      n183 = Index Array(array=w603, index #1=16 ("index"), index #2=27 ("index")) -> (element #1=w609:u8)  [unwired: 1 out]
      n184 = call "MicroPulse - RF slots decoder.vi"("byte array"=w603) -> ("RF Slot status"=w607:string)
      n185 = call "PNDT - assemble version info.vi"("#bytes [2]"=2 ("#bytes"), "start index"=5, "version label"="Hardware", "version bytes"=w603) -> ("version info"=w589:string)  [unwired: 7 in]
      n186 = call "PNDT - assemble version info.vi"("other info"=w589, "#bytes [2]"=4, "start index"=12 ("index"), "version label"="Processor", "version bytes"=w603) -> ("version info"=w587:string)  [unwired: 6 in]
      n187 = call "Pndt byte splitter - U32.vi"("byte U32"=w565, "mask size"=i16 7 ("y"), "shift right"=i16 4 ("y")) -> ("lo"=w563:u32, "hi"=w575:u32)  [unwired: 7 in]
      n188 = call "Pndt byte splitter - U32.vi"("byte U32"=w567, "mask size"=u32 2, "shift right"=i16 4 ("y")) -> ("lo"=w598:u32, "hi"=w570:u32)  [unwired: 7 in]
      n189 = call "Pndt byte splitter - U32.vi"("byte U32"=w604, "mask size"=w611, "shift right"=w611) -> ("lo"=w616:u32, "hi"=w617:u32)  [unwired: 7 in]
      n190 = To Unsigned Byte Integer(number=w598) -> (unsigned 8bit integer=w559:u8)
      n191 = To Unsigned Byte Integer(number=w575) -> (unsigned 8bit integer=w558:u8)
      n192 = To Unsigned Byte Integer(number=w563) -> (unsigned 8bit integer=w556:u8)
      n193 = case shown="Default" w617 {
        selector: w617 -> [_ w630]
        tunnel: ["feature not  available" w629] -> w618
        frame 0, 16 {
        }
        frame Default {
          n194 = Number To Decimal String(number=w630) -> (decimal integer string=w629:string)  [unwired: 1 in]
        }
      }
      n195 = call "MicroPulse - dof decoder.vi"("dof"=w602) -> ("String"=w601:string, "DOF"=w584:T7)  [unwired: 3 in]
      n196 = And(x=w558, y=u8 8) -> (x .and. y?=w552:u8)
      n197 = And(x=w556, y=u8 7) -> (x .and. y?=w554:u8)
      n198 = Join Numbers(hi=w559, lo=w599) -> ((hi.lo)=w572:u16)
      n199 = call "PNDT - assemble version info.vi"("other info"=w587, "#bytes [2]"=4 ("#bytes"), "start index"=28 ("index"), "version label"="Ethernet", "version bytes"=w603) -> ("version info"=w586:string)  [unwired: 6 in]
      n200 = Decrement(x=w554) -> (x-1=w553:u8)
      n201 = Logical Shift(y=i16 -3, x=w552) -> (x << y=w550:u8)
      n202 = call "MicroPulse - system type and serial num decoder.vi"("RST Msg System Type in"=w570, "RST Msg Serial # in"=w572) -> ("System Type Enum"=w561:T6, "System Type String"=w569:string, "Full Serial # out"=w562:u64)  [unwired: 7 in]
      n203 = Join Numbers(hi=w553, lo=w612) -> ((hi.lo)=w577:u16)
      n204 = case shown="FF" w609 {
        tunnel: ["Pass" "Fail"] -> w608
        frame 255 {
        }
        frame Default {
        }
      }
      n205 = case shown="0" w616 {
        tunnel: [i16 40 ("y") i16 60 ("y") i16 70 ("y") _] -> w580
        frame 0 {
        }
        frame 1 {
        }
        frame 3 {
        }
        frame Default {
        }
      }
      n206 = call "MicroPulse - dof decoder.vi"("dof"=w600) -> ("String"=w579:string, "DOF"=w581:T7)  [unwired: 3 in]
      n207 = Bundle By Name(cluster=w564, "Serial No."=w562, "Channels.Extra"=w550, "Channels.PA"=w577, "Channels.Conv"=w571, "System Type"=w561, "Software Versions"=w586, "Data Output Format.Actual"=w584, "Sample Frequency.Default"=w583, "Sample Frequency.Actual"=w582, "Data Output Format.Default"=w581, "DAC Gain"=w580) -> (w578:T5)
      n208 = Format Into String(format string="\nSystem Type = %s\nSerial Number %d\nNo. of Channels = %d\n\rExtra Channels Present = %d\nNo. of PA Channels = %d\nDefault DOF = %s\nActual DOF = %s\nDefault S Freq = %dMHz\nActual S Freq = %dMHz\n\nCUIF ADCs = %s\nDAC Gain = %ddB\nMaster Control = %s\n%s\n\n**Software Versions**\n%s", initial string="---------------\nSystem Status \n---------------", w569, w562, w571, w550, w577, w579, w601, w583, w582, w618, w580, w608, w607, w586) -> (resulting string=w621:string)  [unwired: 1 in, 1 out]
    }
    frame 36 {
      w656 = i16 11 ("y")
      w658 = i16 4 ("y")
      # "GPH Grass-Coupling High"
      n209 = Index Array(array=w652, index #1=1 ("index")) -> (element #1=w650:u8, element #2=w651:u8, element #3=w657:u8, element #4=w645:u8, element #5=w644:u8, element #6=w643:u8, element #7=w642:u8, element #8=w640:u8, element #9=w641:u8)  [unwired: 8 in]
      n210 = Join Numbers(hi=w642, lo=w643) -> ((hi.lo)=w639:u16)
      n211 = Join Numbers(hi=w641, lo=w640) -> ((hi.lo)=w637:u16)
      n212 = Join Numbers(hi=w651, lo=w650) -> ((hi.lo)=w655:u16)
      n213 = Join Numbers(hi=w644, lo=w645) -> ((hi.lo)=w638:u16)
      n214 = Join Numbers(hi=w639, lo=w638) -> ((hi.lo)=w636:u32)
      n215 = call "Pndt byte splitter - U32.vi"("byte U32"=w655, "mask size"=w656, "shift right"=w656) -> ("lo"=w648:u32, "hi"=w649:u32)  [unwired: 7 in]
      n216 = call "Pndt byte splitter - U32.vi"("byte U32"=w657, "mask size"=w658, "shift right"=w658) -> ("lo"=w653:u32, "hi"=w654:u32)  [unwired: 7 in]
      n217 = Increment(x=w648) -> (x+1=w635:u32)
      n218 = call "MicroPulse - dof decoder.vi"("dof"=w653) -> ("String"=w647:string)  [unwired: 3 in, 1 out]
      n219 = case shown="Default" w654 {
        tunnel: ["n.a." "Gate 1" "Gate 2" "Gate 3" "Gate 4"] -> w646
        frame Default {
        }
        frame 1 {
        }
        frame 2 {
        }
        frame 3 {
        }
        frame 4 {
        }
      }
      n220 = Format Into String(format string="\nSweep No. %d\nTest No. %d\nDOF = %s\nGate Mode = %s\nWaveform Integral = %d\nAmplitude = %d", initial string="---------------------------\nGPH Grass-Coupling High\n---------------------------", w649, w635, w647, w646, w636, w637) -> (resulting string=w659:string)  [unwired: 1 in, 1 out]
    }
    frame 37 {
      w693 = i16 11 ("y")
      w695 = i16 4 ("y")
      # "GPL Grass-Coupling Low"
      n221 = Index Array(array=w689, index #1=1 ("index")) -> (element #1=w687:u8, element #2=w688:u8, element #3=w694:u8, element #4=w682:u8, element #5=w681:u8, element #6=w680:u8, element #7=w679:u8, element #8=w677:u8, element #9=w678:u8)  [unwired: 8 in]
      n222 = Join Numbers(hi=w679, lo=w680) -> ((hi.lo)=w676:u16)
      n223 = Join Numbers(hi=w678, lo=w677) -> ((hi.lo)=w674:u16)
      n224 = Join Numbers(hi=w688, lo=w687) -> ((hi.lo)=w692:u16)
      n225 = Join Numbers(hi=w681, lo=w682) -> ((hi.lo)=w675:u16)
      n226 = Join Numbers(hi=w676, lo=w675) -> ((hi.lo)=w673:u32)
      n227 = call "Pndt byte splitter - U32.vi"("byte U32"=w692, "mask size"=w693, "shift right"=w693) -> ("lo"=w685:u32, "hi"=w686:u32)  [unwired: 7 in]
      n228 = call "Pndt byte splitter - U32.vi"("byte U32"=w694, "mask size"=w695, "shift right"=w695) -> ("lo"=w690:u32, "hi"=w691:u32)  [unwired: 7 in]
      n229 = Increment(x=w685) -> (x+1=w672:u32)
      n230 = call "MicroPulse - dof decoder.vi"("dof"=w690) -> ("String"=w684:string)  [unwired: 3 in, 1 out]
      n231 = case shown="Default" w691 {
        tunnel: ["n.a." "Gate 1" "Gate 2" "Gate 3" "Gate 4"] -> w683
        frame Default {
        }
        frame 1 {
        }
        frame 2 {
        }
        frame 3 {
        }
        frame 4 {
        }
      }
      n232 = Format Into String(format string="\nSweep No. %d\nTest No. %d\nDOF = %s\nGate Mode = %s\nWaveform Integral = %d\nAmplitude = %d", initial string="--------------------------\nGPL Grass-Coupling Low\n--------------------------", w686, w672, w684, w683, w673, w674) -> (resulting string=w696:string)  [unwired: 1 in, 1 out]
    }
    frame 38 {
      w729 = i16 11 ("y")
      w731 = i16 4 ("y")
      # "Auto-CAL"
      n233 = Index Array(array=w725, index #1=1 ("index")) -> (element #1=w723:u8, element #2=w724:u8, element #3=w730:u8, element #4=w718:u8, element #5=w717:u8, element #6=w715:u8, element #7=w714:u8, element #8=w711:u8, element #9=w712:u8)  [unwired: 8 in]
      n234 = Join Numbers(hi=w714, lo=w715) -> ((hi.lo)=w713:u16)
      n235 = Join Numbers(hi=w712, lo=w711) -> ((hi.lo)=w710:u16)
      n236 = Join Numbers(hi=w724, lo=w723) -> ((hi.lo)=w728:u16)
      n237 = Join Numbers(hi=w717, lo=w718) -> ((hi.lo)=w716:u16)
      n238 = call "Pndt byte splitter - U32.vi"("byte U32"=w728, "mask size"=w729, "shift right"=w729) -> ("lo"=w721:u32, "hi"=w722:u32)  [unwired: 7 in]
      n239 = call "Pndt byte splitter - U32.vi"("byte U32"=w730, "mask size"=w731, "shift right"=w731) -> ("lo"=w726:u32, "hi"=w727:u32)  [unwired: 7 in]
      n240 = call "MicroPulse - dof decoder.vi"("dof"=w726) -> ("String"=w720:string)  [unwired: 3 in, 1 out]
      n241 = Increment(x=w721) -> (x+1=w709:u32)
      n242 = case shown="Default" w727 {
        tunnel: ["n.a." "Gate 1" "Gate 2" "Gate 3" "Gate 4"] -> w719
        frame Default {
        }
        frame 1 {
        }
        frame 2 {
        }
        frame 3 {
        }
        frame 4 {
        }
      }
      n243 = Format Into String(format string="\nSweep No. %d\nTest No. %d\nDOF = %s\nGate Mode = %s\nAmplitude = %d\nTimebase = %d\nGain = %d", initial string="----------\nAuto-CAL\n----------", w722, w709, w720, w719, w716, w713, w710) -> (resulting string=w732:string)  [unwired: 1 in, 1 out]
    }
    frame 39 {
      w760 = i16 11 ("y")
      # "Set reported Echo Range to zero on echo trigger failure."
      # "ING - Interface echo trigger failure"
      n244 = Unbundle By Name(w745) -> ()  [unwired: 1 out]
      n245 = Index Array(array=w752, index #1=1 ("index")) -> (element #1=w757:u8, element #2=w758:u8, element #3=w755:u8)  [unwired: 2 in]
      n246 = Join Numbers(hi=w758, lo=w757) -> ((hi.lo)=w759:u16)
      n247 = call "Pndt byte splitter - U32.vi"("byte U32"=w759, "mask size"=w760, "shift right"=w760) -> ("lo"=w756:u32, "hi"=w753:u32)  [unwired: 7 in]
      n248 = Increment(x=w756) -> (x+1=w754:u32)
      n249 = disable-structure shown="Enabled" {
        disable-tunnel: [w765 w768] -> w750
        disable-tunnel: w749 -> [w764 w769]
        frame Disabled {
          n250 = Bundle By Name(cluster=w764, "echo range"=u16 0) -> (w765:T9)
        }
        frame Enabled {
          n251 = Bundle By Name(cluster=w769, "ETG"=TRUE) -> (w768:T9)
        }
      }
      n252 = Format Into String(format string=" Test %d/Sweep %d/Chan %d\n", initial string="EGT failure:", w754, w753, w755) -> (resulting string=w747:string, error out=w751:errorcluster)  [unwired: 1 in]
      n253 = Select(t=w747, s=TRUE ("Report Data Msg"), f="") -> (s? t:f=w746:string)
    }
    frame 40 {
      w783 = i16 11 ("y")
      w785 = i16 4 ("y")
      # "LWL Coupling failure"
      n254 = Index Array(array=w780, index #1=1 ("index")) -> (element #1=w778:u8, element #2=w779:u8, element #3=w784:u8)  [unwired: 2 in]
      n255 = Join Numbers(hi=w779, lo=w778) -> ((hi.lo)=w782:u16)
      n256 = call "Pndt byte splitter - U32.vi"("byte U32"=w782, "mask size"=w783, "shift right"=w783) -> ("lo"=w776:u32, "hi"=w777:u32)  [unwired: 7 in]
      n257 = call "Pndt byte splitter - U32.vi"("byte U32"=w784, "mask size"=w785, "shift right"=w785) -> ("lo"=w781:u32)  [unwired: 7 in, 1 out]
      n258 = call "MicroPulse - dof decoder.vi"("dof"=w781) -> ("String"=w775:string)  [unwired: 3 in, 1 out]
      n259 = Increment(x=w776) -> (x+1=w774:u32)
      n260 = Format Into String(format string="\nSweep No. %d\nTest No. %d\nDOF = %s", initial string="----------------------\nLWL Coupling failure\n----------------------", w777, w774, w775) -> (resulting string=w786:string)  [unwired: 1 in, 1 out]
    }
    frame 41 {
      w802 = i16 11 ("y")
      # "Overload failure (1) – 4 Bytes in total:\n<29Hex>\n<Sweep/Test No. lsb >\n<Sweep/Test No. msb >\n<Count of elements saturating during gate>"
      # "Overload failure (1)"
      n261 = Index Array(array=w800, index #1=1 ("index")) -> (element #1=w798:u8, element #2=w799:u8, element #3=w795:u8)  [unwired: 2 in]
      n262 = Join Numbers(hi=w799, lo=w798) -> ((hi.lo)=w801:u16)
      n263 = call "Pndt byte splitter - U32.vi"("byte U32"=w801, "mask size"=w802, "shift right"=w802) -> ("lo"=w796:u32, "hi"=w797:u32)  [unwired: 7 in]
      n264 = Increment(x=w796) -> (x+1=w794:u32)
      n265 = Format Into String(format string="\nSweep No. %d\nTest No. %d\n No. of Saturated Elements = %d", initial string="--------------------\nOverload failure (1)\n--------------------", w797, w794, w795) -> (resulting string=w803:string)  [unwired: 1 in, 1 out]
    }
    frame 42 {
      w823 = i16 11 ("y")
      # "Overload failure (2)\n<2aHex>\n<Total message length count (n+4)>\n<Sweep/Test No. lsb >\n<Sweep/Test No. msb >\n<n Bytes containing a bitwise representation of each channels overload status>"
      # "Overload failure (2)"
      n266 = Index Array(array=w816, index #1=1 ("index")) -> (element #1=w817:u8, element #2=w820:u8, element #3=w821:u8)  [unwired: 2 in]
      n267 = Array Subset(array=w816, index=4) -> (w814:u8[])  [unwired: 1 in]
      n268 = Join Numbers(hi=w821, lo=w820) -> ((hi.lo)=w822:u16)
      n269 = for {
        tunnel: w814 -> [w831] mode=indexing
        tunnel: [w828] -> w813 mode=indexing
        n270 = Number To Hexadecimal String(2:w831) -> (0:w830:string)  [unwired: 1 in]
        n271 = Concatenate Strings(w830, " " ("string")) -> (w828:string)
      }
      n272 = call "Pndt byte splitter - U32.vi"("byte U32"=w822, "mask size"=w823, "shift right"=w823) -> ("lo"=w818:u32, "hi"=w819:u32)  [unwired: 7 in]
      n273 = Increment(x=w818) -> (x+1=w811:u32)
      n274 = Concatenate Strings(w813) -> (w812:string)
      n275 = Format Into String(format string="\nLength = %d bytes\nSweep No. %d\nTest No. %d\nBitwise Overload Status = %s", initial string="--------------------\nOverload failure (2)\n--------------------", w817, w819, w811, w812) -> (resulting string=w824:string)  [unwired: 1 in, 1 out]
    }
    frame 45 {
      # "Add sub-header to header byte"
      # "Universal Header 0x2D"
      n276 = Unbundle By Name(w838) -> ("Report Data Msg"=w840:bool)
      n277 = Index Array(array=w849, index=4) -> (element=w832:u8)
      n278 = Join Numbers(hi=w834, lo=w832) -> ((hi.lo)=w833:u16)
      n279 = case "0x2D Sub-header" shown="46" w832 {
        tunnel: [_ w866 w908 w927 w944 w960 w1014 w1030 w1199 w1228 w1256 w1275 w1298 w1366] -> w842
        tunnel: w849 -> [_ w860 w906 w934 w950 w964 w1018 w1035 w1203 w1229 w1243 w1271 w1293 w1321]
        tunnel: [w854 w895 w899 w928 w943 w974 w1010 w1031 w1194 w1222 w1239 w1269 w1290 w1336] -> w848
        tunnel: w847 -> [w854 w895 w899 w928 w943 w974 w1010 w1032 w1194 w1222 w1239 w1269 w1290 w1313]
        tunnel: w846 -> [w853 w894 w905 w923 w939 w955 w1006 w1034 w1202 w1227 w1236 w1270 w1287 w1308]
        tunnel: [w853 w894 w905 w923 w939 w955 w1006 w1033 w1198 w1226 w1236 w1270 w1287 w1308] -> w845
        tunnel: [_ w867 w909 w926 w942 w958 w1009 w1029 _ _ _ w1276 _ _] -> w844
        tunnel: w840 -> [_ w865 w907 _ _ _ _ _ _ _ _ w1274 _ _]
        tunnel: [TRUE ("Report Data Msg") w865 w907 TRUE ("Report Data Msg") TRUE ("Report Data Msg") TRUE ("Report Data Msg") TRUE ("Report Data Msg") TRUE TRUE ("Report Data Msg") TRUE ("Report Data Msg") TRUE ("Report Data Msg") w1274 TRUE ("Report Data Msg") TRUE ("Report Data Msg")] -> w839
        tunnel: w838 -> [_ w864 _ _ _ _ _ _ _ _ _ _ _ _]
        tunnel: [_ w863 _ _ _ _ _ _ _ _ _ _ _ _] -> w837
        tunnel: [w851 w862 w911 w925 w941 w957 w1007 w1028 w1200 w1223 w1238 w1273 w1288 w1310] -> w836
        tunnel: w835 -> [w851 w861 w910 w925 w941 w957 w1007 w1028 w1200 w1223 w1238 w1272 w1288 w1310]
        frame Default {
        }
        frame 1 {
          w875 = u8 26 ("header (1A)")
          w878 = u32 12 ("y")
          w890 = i16 11 ("y")
          # "Data Message with EGT Range message in FMC\nTo support FMC mode individual channel echo gate trigger the following messages are used.\n< Universal Header 0x2d><count lsb><count tsb><count msb><Sub-header 0x01>\n<Sweep No./Test No. lsb> <Sweep No./Test No. msb><dof ><Channel >\n<Echo range lsb><Echo range msb><Spare> <amp 1>….. <amp n >\n\nWhere:\nHeader: universal header 0x2d\nCount: 24 bit total data length count\nSub-header byte: 0x01 = FMC Ascan\nSweep/Test No: 16 bits. Bottom 11 bits Test No. Top 5 bits sweep No.\ndof: data format\nChannel: Normally 0, except in full matrix capture tests it is used to indicate the channel number\nEcho Range: Range of the interface echo from the start of the interface echo gate.\nSpare Not used.\namp: In 8 bit Modes, for Ascan = amplitudes of digitised signal. In greater than 8 bit modes, the amplitudes are least significant byte first."
          # "FMC Ascan"
          n280 = call "Pndt 1-4 byte combiner.vi"("#bytes"=3, "start index [0]"=1, "[U8] count bytes"=w860) -> ("U32"=w863:u32)
          n281 = Subtract(x=w863, y=w878) -> (x-y=w877:u32)
          n282 = Index Array(array=w860, index #1=5 ("index")) -> (element #1=w887:u8, element #2=w888:u8, element #3=w883:u8, element #4=w855:u8, element #5=w882:u8, element #6=w881:u8)  [unwired: 5 in]
          n283 = Array Subset(array=w860, index=w878, length=w877) -> (w874:u8[])
          n284 = Join Numbers(hi=w881, lo=w882) -> ((hi.lo)=w879:u16)
          n285 = Join Numbers(hi=w888, lo=w887) -> ((hi.lo)=w889:u16)
          n286 = call "Pndt byte splitter - U32.vi"("byte U32"=w889, "mask size"=w890, "shift right"=w890) -> ("lo"=w886:u32, "hi"=w880:u32)  [unwired: 7 in]
          n287 = case shown="Default" w855 {
            selector: w855 -> [_ w898]
            tunnel: ["n.a." w897] -> w884
            frame 0 {
            }
            frame Default {
              n288 = Format Into String(w898) -> (resulting string=w897:string)  [unwired: 3 in, 1 out]
            }
          }
          n289 = call "MicroPulse - dof decoder.vi"("dof"=w883) -> ("String"=w885:string, "DOF"=w856:T7)  [unwired: 3 in]
          n290 = Unbundle By Name(w864) -> ("Sub Sampling"=w871:T2, "Scan Reset"=w857:bool)
          n291 = Increment(x=w886) -> (x+1=w869:u32)
          n292 = call "PNDT - waveform decoder.vi"("header (1A)"=w875, "[U8]"=w874, "DOF"=w856) -> ("scan data"=w876:u16[])  [unwired: 5 in, 3 out]
          n293 = call "PNDT - subsampling data reduction.vi"("sub-sampling"=w871, "header (1A)"=w875, "data set"=w876) -> ("reduced data set"=w872:u16[], "scan length"=w873:i32)  [unwired: 7 in]
          n294 = To Long Integer(number=w869) -> (32bit integer=w868:i32)
          n295 = call "PNDT - test number to scan index.vi"("reset"=w857, "test no."=w868) -> ("scan index"=w870:i32)  [unwired: 2 in, 1 out]
          n296 = Format Into String(format string="\nSweep No. %d\nTest No. %d\nDOF: %s\nChannel No. %s\nEcho Range: %d", initial string="------------\nFMC Ascan\n------------", w880, w869, w885, w884, w879) -> (resulting string=w866:string, error out=w867:errorcluster)  [unwired: 1 in]
          n297 = Bundle By Name(cluster=w861, "Sweep No."=w880, "Test No."=w868, "scan index"=w870, "DOF"=w856, "Channel No."=w855, "echo range"=w879, "scan length"=w873, "scan data"=w872) -> (w862:T9)
        }
        frame 2 {
          w919 = i16 11 ("y")
          # "To support the reporting of the interface echo range for Multi-gate modes:\n\n< Universal Header 0x2d><count lsb><count tsb><count msb><Sub-header 0x02>\n<Sweep/Test No. lsb ><Sweep/Test No. msb ><dof><Echo Range lsb >\n<Echo Range msb ><spare 0><spare 0>\n \nWhere:\nHeader: universal header 0x2d\nCount: 24 bit total data length count\nSub-header byte: 0x02 = EGT range\nSweep/Test No: 16 bits. Bottom 11 bits Test No. Top 5 bits sweep No.\ndof: data format\nEcho Range: Echo Range is reported at the sample frequency and from the time of the initial pulse\nSpare Not used and set to 0"
          # "Interface Echo Range Message"
          n298 = Index Array(array=w906, index #1=5 ("index")) -> (element #1=w916:u8, element #2=w917:u8, element #3=w914:u8, element #4=w912:u8, element #5=w913:u8)  [unwired: 6 in, 2 out]
          n299 = Join Numbers(hi=w913, lo=w912) -> ((hi.lo)=w900:u16)
          n300 = Join Numbers(hi=w917, lo=w916) -> ((hi.lo)=w918:u16)
          n301 = call "Pndt byte splitter - U32.vi"("byte U32"=w918, "mask size"=w919, "shift right"=w919) -> ("lo"=w902:u32, "hi"=w904:u32)  [unwired: 7 in]
          n302 = Increment(x=w902) -> (x+1=w903:u32)
          n303 = call "MicroPulse - dof decoder.vi"("dof"=w914) -> ("String"=w915:string)  [unwired: 3 in, 1 out]
          n304 = Format Into String(format string="\nTest No. %d\nSweep No. %d\nDOF: %s\nEcho Range: %d", initial string="-----------------------\nEGT: Echo Gate Range\n-----------------------", w903, w904, w915, w900) -> (resulting string=w908:string, error out=w909:errorcluster)  [unwired: 1 in]
          n305 = Bundle By Name(cluster=w910, "ETG"=FALSE, "echo range"=w900) -> (w911:T9)
        }
        frame 3 {
          # "STX (Enter Idle Mode)\n\nPurpose: To enter idle mode with no test displayed.\n\nFormat: STX [option]\n\nDescription: This command is useful for suspending pulser activity.\nParameters: [option] : If omitted all test activity is stopped and any remaining test data is sent to the host.\n= 1. All test activity is stopped, the contents of the data buffer are erased and a message is sent to indicate completion. For the format of the output message see the MicroPulse Output Messages Section. Prior to the STX 1 complete message MicroPulse may also send a series of header 0 messages (single byte). This is to ensure that the last data set has been completed prior to the STX 1 complete message and maintain message synchronisation with the host. Header 0 messages should be discarded."
          # "STX 1 completion message"
          n306 = Index Array(array=w934, index=5) -> (element=w933:u8)
          n307 = case shown="0" w933 {
            tunnel: ["Buffer Cleared Successfully" "Instrument buffer NOT cleared." "Only partial buffer clear" "Message not supported"] -> w929
            frame 0 {
            }
            frame 1 {
            }
            frame 2 {
            }
            frame Default {
            }
          }
          n308 = Format Into String(format string="\n%s\n", initial string="------------------\nSTX 1 Completed\n------------------", w929) -> (resulting string=w927:string, error out=w926:errorcluster)  [unwired: 1 in]
        }
        frame 4 {
          # "Sync Mode Error Msg - SYNC"
          n309 = Index Array(array=w950, index=5) -> (element=w949:u8)
          n310 = case shown="2" w949 {
            tunnel: ["Pass" "Master SYNC error" "Slave SYNC error" "Message not supported"] -> w945
            frame 0 {
            }
            frame 1 {
            }
            frame 2 {
            }
            frame Default {
            }
          }
          n311 = Format Into String(format string="\n%s", initial string="------------------\nSYNC Mode Error\n------------------", w945) -> (resulting string=w944:string, error out=w942:errorcluster)  [unwired: 1 in]
        }
        frame 48 {
          # "SCHK - Detailed Report Msg"
          n312 = Index Array(array=w964, index #1=5 ("index")) -> (element #1=w975:u8, element #2=w977:u8, element #3=w973:u8, element #4=w971:u8, element #5=w972:u8, element #6=w969:u8, element #7=w968:u8)  [unwired: 6 in]
          n313 = Join Numbers(hi=w972, lo=w971) -> ((hi.lo)=w970:u16)
          n314 = Join Numbers(hi=w968, lo=w969) -> ((hi.lo)=w967:u16)
          n315 = Array Subset(array=w964, index=12, length=48) -> (w963:u8[])
          n316 = for {
            tunnel: w963 -> [w995]
            tunnel: string[] ["0dB", "+2dB", "-6dB", "-12dB", "-18dB", "-24dB"] -> [w984] mode=indexing
            tunnel: [w985] -> w959 mode=indexing
            i -> [w987]
            w986 = 8 ("length")
            n317 = Multiply(x=w987, y=w986) -> (x*y=w988:i32)
            n318 = Array Subset(array=w995, index=w988, length=w986) -> (w989:u8[])
            n319 = Index Array(array=w989) -> (element #1=w996:u8, element #3=w994:u8, element #5=w993:u8, element #7=w991:u8, element #8=w992:u8)  [unwired: 8 in, 3 out]
            n320 = Concatenate Strings("\nGain Setting: " ("string"), w984, "\n-----------------\n" ("string")) -> (w983:string)
            n321 = Join Numbers(hi=w992, lo=w991) -> ((hi.lo)=w990:u16)
            n322 = Format Into String(format string="Positive Limit: %d\nNegative Limit: %d\nAmplitude: %d\nTimebase: %d\n", initial string=w983, w996, w994, w993, w990) -> (resulting string=w985:string)  [unwired: 1 in, 1 out]
          }
          n323 = case shown="4" w977 {
            tunnel: ["Pass" "On Auto CAL no peak found in gate" "Even at minimum Pulser Volts, reference signal is too high" "Reference peak too low" "Reference peak found but too little gain for linearity checks" "Reference peak found but too much gain for linearity checks" "Linearity check outside limits" "Message not supported"] -> w976
            tunnel: w973 -> [_ _ _ _ _ _ _ _]
            frame 0 {
            }
            frame 1 {
            }
            frame 2 {
            }
            frame 3 {
            }
            frame 4 {
            }
            frame 5 {
            }
            frame 6 {
            }
            frame Default {
            }
          }
          n324 = Format Into String(format string=" \nPA Channel No: %d\nResult: %s\nPulser Voltage: %d\nReference Gain (80\\%): %d\n", initial string="-----------------------\nSCHK Detailed Report\n-----------------------", w975, w976, w970, w967) -> (resulting string=w978:string, error out=w958:errorcluster)  [unwired: 1 in]
          n325 = Concatenate Strings(w978, w959) -> (w960:string)
        }
        frame 49 {
          # "SCHK - Simple Report Msg"
          n326 = Index Array(array=w1018, index #1=5 ("index")) -> (element #1=w1011:u8, element #2=w1013:u8)  [unwired: 1 in]
          n327 = case shown="1" w1013 {
            tunnel: ["Pass" "On Auto CAL no peak found in gate" "Even at minimum Pulser Volts, reference signal is too high" "Reference peak too low" "Reference peak found but too little gain for linearity checks" "Reference peak found but too much gain for linearity checks" "Linearity check outside limits" "Message not supported"] -> w1012
            frame 0 {
            }
            frame 1 {
            }
            frame 2 {
            }
            frame 3 {
            }
            frame 4 {
            }
            frame 5 {
            }
            frame 6 {
            }
            frame Default {
            }
          }
          n328 = Format Into String(format string="\n PA Channel No: %d\nResult: %s", initial string="-----------------------\nSCHK Report Message\n-----------------------", w1011, w1012) -> (resulting string=w1014:string, error out=w1009:errorcluster)  [unwired: 1 in]
        }
        frame 64 {
          # "LLC message\nThe LLC message is generated in response to a STA command and gives the current location for all axes.\n\n(32 Bit mode)\n< Universal Header 0x2d><count lsb><count tsb><count msb>\n< LLC Sub-header 0x40><status><K1><K2><K3><K4><Info>\nWhere:\nHeader: Universal header 0x2d\nCount: 24 bit total data length count\nSub-header: The LLC sub-header 0x40\nStatus: Status Byte (reflection of the optional parameter in STA)\nKn: Four byte location of axis n, least significant first.\nInfo: Four Bytes normally set to 0xffffffff, but in moving inspection modes can be configured to give information on the number of Bytes left in the system buffer when the test was fired (Status = 1)."
          # "LLC axis status (32b)"
          n329 = Index Array(array=w1035, index=5) -> (element=w1038:u8)
          n330 = case shown="0, 1, F0" w1038 {
            selector: w1038 -> [_ w1044 w1076 w1096 w1125 w1134 w1160 w1178 w1190]
            tunnel: w1035 -> [_ w1049 w1083 w1103 w1123 w1141 w1158 w1172 w1186]
            tunnel: [w1040 w1056 w1078 w1098 w1117 w1136 w1162 w1177 w1192] -> w1033
            tunnel: [_ w1055 w1077 w1097 w1126 w1135 w1161 w1179 w1183] -> w1030
            tunnel: w1034 -> [w1042 w1053 w1074 w1093 w1117 w1132 w1152 w1177 w1192]
            tunnel: w1032 -> [w1043 w1052 w1073 w1094 w1116 w1131 w1151 w1171 w1193]
            tunnel: [w1043 w1052 w1073 w1094 w1115 w1131 w1151 w1170 w1193] -> w1031
            tunnel: "--------------------\nLLC MESSAGE (32b)\n--------------------" -> [_ w1046 w1072 w1092 w1111 w1130 w1150 w1166 w1182]
            tunnel: [w1039 w1045 w1071 w1091 w1110 w1129 w1149 w1164 w1181] -> w1029
            frame Default {
              n331 = Variant To Data(type=T3 {"Axis Positions"={"Axis 1"=0, "Axis 2"=0, "Axis 3"=0, "Axis 4"=0, "Status"=0}, "MPE Settings"={"Axis 1"=0, "Axis 2"=0, "Axis 3"=0, "Axis 4"=0}, "BKL Settings"={"Axis 1"=0, "Axis 2"=0, "Axis 3"=0, "Axis 4"=0}, "SPA Settings"={"Axis 1"=0, "Axis 2"=0, "Axis 3"=0, "Axis 4"=0}, "IP"={"Axis No."=0, "Location"=0}, "MIP"={"Axis No."=0, "Location"=0}, "IO Levels"={"Inputs: 15-8"=0, "Inputs: 7-0"=0, "Outputs: 15-8"=0, "Outputs: 7-0"=0}} ("Axis Status"), Variant=w1042) -> (data=w1040:T3, error out=w1039:errorcluster)  [unwired: 1 in]
            }
            frame 0, 1, 240 {
              w1061 = 4 ("#bytes")
              # "STA/STS 0 - Axis Positions"
              n332 = call "Pndt 1-4 byte combiner.vi"("#bytes"=4, "start index [0]"=22, "[U8] count bytes"=w1049) -> ("U32"=w1047:u32)
              n333 = call "Pndt 1-4 byte combiner.vi"("#bytes"=w1061, "start index [0]"=6, "[U8] count bytes"=w1049) -> ("U32"=w1060:u32)
              n334 = call "Pndt 1-4 byte combiner.vi"("#bytes"=w1061, "start index [0]"=10, "[U8] count bytes"=w1049) -> ("U32"=w1059:u32)
              n335 = call "Pndt 1-4 byte combiner.vi"("#bytes"=w1061, "start index [0]"=14, "[U8] count bytes"=w1049) -> ("U32"=w1058:u32)
              n336 = call "Pndt 1-4 byte combiner.vi"("#bytes"=w1061, "start index [0]"=18, "[U8] count bytes"=w1049) -> ("U32"=w1057:u32)
              n337 = case shown="Default" w1047 {
                tunnel: [w1068 _] -> w1048
                tunnel: w1047 -> [w1067 _]
                frame Default {
                  n338 = Format Into String(format string="Bytes left in Buffer = %d", w1067) -> (resulting string=w1068:string)  [unwired: 2 in, 1 out]
                }
                frame 0, -1 {
                }
              }
              n339 = Format Into String(format string="\nStatus %x\n%s\nAxis 1: %d\nAxis 2: %d\nAxis 3: %d\nAxis 4: %d\n%s", initial string=w1046, w1044, "Axis Positions (counts)", w1060, w1059, w1058, w1057, w1048) -> (resulting string=w1055:string, error out=w1045:errorcluster)  [unwired: 1 in]
              n340 = Bundle By Name(cluster=w1053, "Axis Positions.Status"=w1044, "Axis Positions.Axis 1"=w1060, "Axis Positions.Axis 2"=w1059, "Axis Positions.Axis 3"=w1058, "Axis Positions.Axis 4"=w1057) -> (w1056:T3)
            }
            frame 241 {
              w1084 = 4 ("#bytes")
              # "STS 1 - MPE Settings"
              n341 = call "Pndt 1-4 byte combiner.vi"("#bytes"=w1084, "start index [0]"=6, "[U8] count bytes"=w1083) -> ("U32"=w1082:u32)
              n342 = call "Pndt 1-4 byte combiner.vi"("#bytes"=w1084, "start index [0]"=10, "[U8] count bytes"=w1083) -> ("U32"=w1081:u32)
              n343 = call "Pndt 1-4 byte combiner.vi"("#bytes"=w1084, "start index [0]"=14, "[U8] count bytes"=w1083) -> ("U32"=w1080:u32)
              n344 = call "Pndt 1-4 byte combiner.vi"("#bytes"=w1084, "start index [0]"=18, "[U8] count bytes"=w1083) -> ("U32"=w1079:u32)
              n345 = Format Into String(format string="\nStatus %x\n%s\nAxis 1: %d\nAxis 2: %d\nAxis 3: %d\nAxis 4 %d", initial string=w1072, w1076, "MPE Settings", w1082, w1081, w1080, w1079) -> (resulting string=w1077:string, error out=w1071:errorcluster)  [unwired: 1 in]
              n346 = Bundle By Name(cluster=w1074, "MPE Settings.Axis 1"=w1082, "MPE Settings.Axis 2"=w1081, "MPE Settings.Axis 3"=w1080, "MPE Settings.Axis 4"=w1079, "Axis Positions.Status"=u8 255) -> (w1078:T3)
            }
            frame 242 {
              w1104 = 4 ("#bytes")
              # "STS 2 - BKL Settings"
              n347 = call "Pndt 1-4 byte combiner.vi"("#bytes"=w1104, "start index [0]"=6, "[U8] count bytes"=w1103) -> ("U32"=w1102:u32)
              n348 = call "Pndt 1-4 byte combiner.vi"("#bytes"=w1104, "start index [0]"=10, "[U8] count bytes"=w1103) -> ("U32"=w1101:u32)
              n349 = call "Pndt 1-4 byte combiner.vi"("#bytes"=w1104, "start index [0]"=14, "[U8] count bytes"=w1103) -> ("U32"=w1100:u32)
              n350 = call "Pndt 1-4 byte combiner.vi"("#bytes"=w1104, "start index [0]"=18, "[U8] count bytes"=w1103) -> ("U32"=w1099:u32)
              n351 = Format Into String(format string="\nStatus %x\n%s\nAxis 1: %d\nAxis 2: %d\nAxis 3: %d\nAxis 4 %d", initial string=w1092, w1096, "BKL Settings", w1102, w1101, w1100, w1099) -> (resulting string=w1097:string, error out=w1091:errorcluster)  [unwired: 1 in]
              n352 = Bundle By Name(cluster=w1093, "BKL Settings.Axis 1"=w1102, "BKL Settings.Axis 2"=w1101, "BKL Settings.Axis 3"=w1100, "BKL Settings.Axis 4"=w1099, "Axis Positions.Status"=u8 255) -> (w1098:T3)
            }
            frame 244 {
              # "STS 20 - System Temperatures"
              n353 = Index Array(array=w1123, index #1=6 ("index"), index #2=8 ("index"), index #3=10 ("index"), index #4=12 ("index")) -> (element #1=w1121:u8, element #2=w1120:u8, element #3=w1119:u8, element #4=w1118:u8)
              n354 = Format Into String(format string="Status %x\n\n%s\nSystem %d degC\nMicroprocessor %d degC\nSlave System %d degC\nSlave Microprocessor %d degC", initial string=w1111, w1125, "---------------------------\nInstrument Temperatures\n---------------------------", w1121, w1120, w1119, w1118) -> (resulting string=w1126:string, error out=w1110:errorcluster)  [unwired: 1 in]
              n355 = Bundle By Name(cluster=w1116, "Temperatures.System"=w1121, "Temperatures.Processor"=w1120, "Temperatures.Slave Sys"=w1119, "Temperatures.Slave Proc"=w1118) -> (w1115:T5)
            }
            frame 245 {
              w1142 = 4 ("#bytes")
              # "STS 5 - SPA Settings"
              n356 = call "Pndt 1-4 byte combiner.vi"("#bytes"=w1142, "start index [0]"=6, "[U8] count bytes"=w1141) -> ("U32"=w1140:u32)
              n357 = call "Pndt 1-4 byte combiner.vi"("#bytes"=w1142, "start index [0]"=10, "[U8] count bytes"=w1141) -> ("U32"=w1139:u32)
              n358 = call "Pndt 1-4 byte combiner.vi"("#bytes"=w1142, "start index [0]"=14, "[U8] count bytes"=w1141) -> ("U32"=w1138:u32)
              n359 = call "Pndt 1-4 byte combiner.vi"("#bytes"=w1142, "start index [0]"=18, "[U8] count bytes"=w1141) -> ("U32"=w1137:u32)
              n360 = Format Into String(format string="\nStatus %x\n%s\nAxis 1: %d\nAxis 2: %d\nAxis 3: %d\nAxis 4 %d", initial string=w1130, w1134, "SPA Settings", w1140, w1139, w1138, w1137) -> (resulting string=w1135:string, error out=w1129:errorcluster)  [unwired: 1 in]
              n361 = Bundle By Name(cluster=w1132, "SPA Settings.Axis 1"=w1140, "SPA Settings.Axis 2"=w1139, "SPA Settings.Axis 3"=w1138, "SPA Settings.Axis 4"=w1137, "Axis Positions.Status"=u8 255) -> (w1136:T3)
            }
            frame 246 {
              # "STS 6 - I/O Line Status"
              n362 = Index Array(array=w1158, index #1=6 ("index")) -> (element #1=w1156:u8, element #2=w1155:u8, element #3=w1154:u8, element #4=w1153:u8)  [unwired: 4 in, 1 out]
              n363 = Format Into String(format string="\nStatus %x\n%s\nInputs 15-8: %b\nInputs 7-0: %b\nOutputs 15-8: %b\nOutputs 7-0: %b", initial string=w1150, w1160, "I/O Status", w1156, w1155, w1154, w1153) -> (resulting string=w1161:string, error out=w1149:errorcluster)  [unwired: 1 in]
              n364 = Bundle By Name(cluster=w1152, "IO Levels.Inputs: 15-8"=w1156, "IO Levels.Inputs: 7-0"=w1155, "IO Levels.Outputs: 15-8"=w1154, "IO Levels.Outputs: 7-0"=w1153, "Axis Positions.Status"=u8 255) -> (w1162:T3)
            }
            frame 247 {
              w1165 = 4 ("index")
              # "STS 7 - Uptimes since last reset"
              n365 = call "Pndt 1-4 byte combiner.vi"("#bytes"=w1165, "start index [0]"=14 ("index"), "[U8] count bytes"=w1172) -> ("U32"=w1167:u32)
              n366 = call "Pndt 1-4 byte combiner.vi"("#bytes"=w1165, "start index [0]"=6 ("index"), "[U8] count bytes"=w1172) -> ("U32"=w1169:u32)
              n367 = call "Pndt 1-4 byte combiner.vi"("#bytes"=w1165, "start index [0]"=10 ("index"), "[U8] count bytes"=w1172) -> ("U32"=w1168:u32)
              n368 = call "MicroPulse - uptime msg assembly.vi"("SRST"=w1167, "RST"=w1168, "Uptime"=w1169) -> ("String"=w1173:string)  [unwired: 8 in]
              n369 = Format Into String(format string="\nStatus %x\n%s", initial string=w1166, w1178, w1173) -> (resulting string=w1179:string, error out=w1164:errorcluster)  [unwired: 1 in]
              n370 = Bundle By Name(cluster=w1171, "Uptimes.since Power"=w1169, "Uptimes.since RSTS"=w1168, "Uptimes.since SRST"=w1167) -> (w1170:T5)
            }
            frame 248 {
              # "STS 8 - System Information (System Status)"
              n371 = Array Subset(array=w1186, index=6) -> (w1184:u8[])  [unwired: 1 in]
              n372 = Number To Hexadecimal String(1:u8 2 ("width (-)"), 2:w1184) -> (0:w1189:string[])
              n373 = Concatenate Strings(w1189) -> (w1188:string)
              n374 = Format Into String(format string="\nStatus %x\nSys Info %s", initial string=w1182, w1190, w1188) -> (resulting string=w1183:string, error out=w1181:errorcluster)  [unwired: 1 in]
            }
          }
        }
        frame 65 {
          # "copy location into LLC record"
          # "LCI message\nThe LCI message is output during a moving inspection mode. It precedes any data from an inspection point and gives the actual location of that inspection point.\n\n(32 Bit mode)\n< Universal Header 0x2d ><count lsb><count tsb><count msb>\n< LCI Sub-header 0x41><axis><K axis>\nWhere:\nHeader: Universal header 0x2d\nCount: 24 bit total data length count\nSub-header: The LCI sub-header 0x41\naxis: Axis number n\nKn: Four byte location of axis n, least significant first."
          # "LCI inspection point location (32b)"
          n375 = Index Array(array=w1203, index=5) -> (element=w1197:u8)
          n376 = call "Pndt 1-4 byte combiner.vi"("#bytes"=4, "start index [0]"=6, "[U8] count bytes"=w1203) -> ("U32"=w1196:u32)
          n377 = Format Into String(format string="\nAxis No. %d\nInspection Point Location: %d", initial string="------------------\nLCI MESSAGE (32b)\n------------------", w1197, w1196) -> (resulting string=w1199:string)  [unwired: 1 in, 1 out]
          n378 = Bundle By Name(cluster=w1202, "IP.Axis No."=w1197, "IP.Location"=w1196) -> (w1201:T3)
          n379 = case shown="4" w1197 {
            tunnel: w1201 -> [w1209 w1212 w1215 w1218 w1221]
            tunnel: [w1209 w1211 w1214 w1217 w1220] -> w1198
            tunnel: w1196 -> [_ w1210 w1213 w1216 w1219]
            frame 0, Default {
              # "Error - Do nothing"
            }
            frame 1 {
              n380 = Bundle By Name(cluster=w1212, "Axis Positions.Axis 1"=w1210) -> (w1211:T3)
            }
            frame 2 {
              n381 = Bundle By Name(cluster=w1215, "Axis Positions.Axis 2"=w1213) -> (w1214:T3)
            }
            frame 3 {
              n382 = Bundle By Name(cluster=w1218, "Axis Positions.Axis 3"=w1216) -> (w1217:T3)
            }
            frame 4 {
              n383 = Bundle By Name(cluster=w1221, "Axis Positions.Axis 4"=w1219) -> (w1220:T3)
            }
          }
        }
        frame 66 {
          # "LCA message\n\nThe LCA message is used to indicate a missed inspection point. The format of this message is as shown above, unless the message is generated due to the MicroPulse buffer being full. In this case the LCA has the top bit of the axis byte is set to 1.\n\n(32 Bit mode)\n< Universal Header 0x2d ><count lsb><count tsb><count msb>\n< LCA Sub-header 0x42><axis><K axis>\nWhere:\nHeader: Universal header 0x2d\nCount: 24 bit total data length count\nSub-header: The LCA sub-header 0x42\naxis: Axis number n\nKn: Four byte location of axis n, least significant first."
          # "LCA missed inspection point (32b)"
          n384 = call "Pndt 1-4 byte combiner.vi"("#bytes"=4, "start index [0]"=6, "[U8] count bytes"=w1229) -> ("U32"=w1235:u32)
          n385 = Index Array(array=w1229, index=5) -> (element=w1225:u8)
          n386 = Format Into String(format string="\nAxis No. %d\nMissed Inspection Point:  %d", initial string="---------------------\nLCA MESSAGE (32b)\n---------------------", w1225, w1235) -> (resulting string=w1228:string)  [unwired: 1 in, 1 out]
          n387 = Bundle By Name(cluster=w1227, "MIP.Axis No."=w1225, "MIP.Location"=w1235) -> (w1226:T3)
        }
        frame 67 {
          w1242 = u32 8 ("y")
          # "CER: Extended Error Msg"
          n388 = Index Array(array=w1243, index #1=5 ("index")) -> (element #1=w1259:u8, element #2=w1253:u8, element #3=w1252:u8)  [unwired: 2 in]
          n389 = call "Pndt 1-4 byte combiner.vi"("#bytes"=3 ("index"), "start index [0]"=1 ("index"), "[U8] count bytes"=w1243) -> ("U32"=w1245:u32)
          n390 = Join Numbers(hi=w1252, lo=w1253) -> ((hi.lo)=w1251:u16)
          n391 = case shown="8" w1259 {
            tunnel: ["Argument conflict " "Unrecognised command " "Argument outside standard limits " "System over temperature " "EHT supply error " "Slave system error " "Parallel channel or Phased Array interface trigger mode error " "Conventional channel VPN mode error "] -> w1255
            frame 0, Default {
            }
            frame 1, 3 {
            }
            frame 2 {
            }
            frame 4 {
            }
            frame 5 {
            }
            frame 6 {
            }
            frame 7 {
            }
            frame 8 {
            }
          }
          n392 = Subtract(x=w1245, y=w1242) -> (x-y=w1244:u32)
          n393 = Array Subset(array=w1243, index=w1242, length=w1244) -> (w1241:u8[])
          n394 = Byte Array To String(unsigned byte array=w1241) -> (string=w1240:string)
          n395 = Number To Decimal String(number=w1251) -> (decimal integer string=w1250:string)  [unwired: 1 in]
          n396 = Concatenate Strings("at character position ", w1250) -> (w1248:string)
          n397 = Concatenate Strings(w1255, w1248) -> (w1254:string)
          n398 = Format Into String(format string="\n%s\n%s", initial string="-------------------\nCER: Ext Error Msg\n-------------------", w1254, w1240) -> (resulting string=w1256:string)  [unwired: 1 in, 1 out]
        }
        frame 68 {
          # "PRF Cycle Time"
          n399 = call "Pndt 1-4 byte combiner.vi"("#bytes"=3 ("index"), "start index [0]"=5 ("index"), "[U8] count bytes"=w1271) -> ("U32"=w1284:u32)
          n400 = To Double Precision Float(number=w1284) -> (double precision float=w1282:dbl)
          n401 = call <vilib>:"Mean PtByPt.vi"("x"=w1282, "sample length"=100) -> ("mean"=w1281:dbl)  [unwired: 2 in, 1 out]
          n402 = Reciprocal(x=6.4e-07 ("y")) -> (1/x=w1279:dbl)
          n403 = Divide(x=w1279, y=w1281) -> (x/y=w1277:dbl)
          n404 = Format Into String(format string="PRF = %d", w1277) -> (resulting string=w1275:string, error out=w1276:errorcluster)  [unwired: 2 in]
          n405 = Bundle By Name(cluster=w1272, "PRF"=w1277) -> (w1273:T9)
        }
        frame 69 {
          (unwired) "-\u001c\u0000\u0000E\u0001\u0000\u0004È\u0014\u0000\u0001\u0007°\u0000\u0000\u0000 \u0000\u0000\u0000°\u0000\u0000\u0000\u0000Zþ"  # Example error log
          # "Error Log Report Message"
          n406 = Index Array(array=w1293, index #1=5 ("index")) -> (element #1=w1295:u8, element #2=w1294:u8, element #3=w1296:u8)  [unwired: 2 in]
          n407 = Join Numbers(hi=w1294, lo=w1295) -> ((hi.lo)=w1291:u16)
          n408 = case shown="4" w1296 {
            tunnel: ["Error Log Disabled" "Error Log Enabled" "Message not supported"] -> w1297
            frame 0 {
            }
            frame 4 {
            }
            frame Default {
            }
          }
          n409 = call "MicroPulse - decode error log report.vi"("data"=w1293, "No. of Logs"=w1291) -> ("error report"=w1292:string)  [unwired: 9 in]
          n410 = Format Into String(format string="\nNo. of Log Messages = %d\n%s\n\n%s", initial string="-----------------\nError Log Report\n-----------------", w1291, w1297, w1292) -> (resulting string=w1298:string)  [unwired: 1 in, 1 out]
        }
        frame 70 {
          w1348 = 4 ("#bytes [2]")
          # "Only for LTPA model  and above.\n(limited on MP5)"
          # "System Information"
          n411 = Index Array(array=w1321, index=5) -> (element=w1337:u8)
          n412 = Index Array(array=w1321, index #1=96 ("index"), index #5=103 ("index")) -> (element #1=w1326:u8, element #2=w1325:u8, element #3=w1324:u8, element #4=w1323:u8, element #5=w1322:u8)  [unwired: 3 in]
          n413 = call "Pndt 1-4 byte combiner.vi"("#bytes"=2 ("index"), "start index [0]"=6 ("index"), "[U8] count bytes"=w1321) -> ("U32"=w1307:u32)
          n414 = call "Pndt 1-4 byte combiner.vi"("#bytes"=2 ("index"), "start index [0]"=8 ("index"), "[U8] count bytes"=w1321) -> ("U32"=w1334:u32)
          n415 = call "Pndt 1-4 byte combiner.vi"("#bytes"=2 ("index"), "start index [0]"=10 ("index"), "[U8] count bytes"=w1321) -> ("U32"=w1333:u32)
          n416 = call "Pndt 1-4 byte combiner.vi"("#bytes"=2 ("index"), "start index [0]"=12 ("index"), "[U8] count bytes"=w1321) -> ("U32"=w1332:u32)
          n417 = call "PNDT - assemble version info.vi"("start index"=14, "version label"="Hardware", "version bytes"=w1321) -> ("version info"=w1315:string)  [unwired: 8 in]
          n418 = Index Array(array=w1321, index #1=16 ("index")) -> (element #1=w1331:u8, element #2=w1330:u8, element #3=w1354:u8, element #4=w1352:u8)  [unwired: 3 in]
          n419 = call "Pndt 1-4 byte combiner.vi"("#bytes"=3 ("index"), "start index [0]"=28 ("index"), "[U8] count bytes"=w1321) -> ("U32"=w1344:u32)
          n420 = call "PNDT - assemble version info.vi"("other info"=w1315, "#bytes [2]"=w1348, "start index"=20, "version label"="Processor", "version bytes"=w1321) -> ("version info"=w1314:string)  [unwired: 6 in]
          n421 = case shown="0" w1344 {
            tunnel: [_ "none" "System flash fail/re-read" "System flash no configured" "System I/O interface fail" "System PSU fail" "Conventional ADC fail"] -> w1311
            frame Default {
            }
            frame 0 {
            }
            frame 1 {
            }
            frame 2 {
            }
            frame 4 {
            }
            frame 8 {
            }
            frame 16 {
            }
          }
          n422 = call "Pndt 1-4 byte combiner.vi"("#bytes"=3 ("index"), "start index [0]"=2 ("index"), "[U8] count bytes"=w1321) -> ("U32"=w1339:u32)
          n423 = call "PNDT - assemble version info.vi"("other info"=w1314, "#bytes [2]"=w1348, "start index"=24, "version label"="Ethernet", "version bytes"=w1321) -> ("version info"=w1312:string)  [unwired: 6 in]
          n424 = call "MicroPulse - dof decoder.vi"("dof"=w1354) -> ("String"=w1353:string, "DOF"=w1329:T7)  [unwired: 3 in]
          n425 = call "MicroPulse - system type and serial num decoder.vi"("Extended Msg?"=TRUE, "RST Msg System Type in"=w1337, "RST Msg Serial # in"=w1307) -> ("System Type Enum"=w1335:T6, "System Type String"=w1338:string, "Full Serial # out"=w1306:u64)  [unwired: 6 in]
          n426 = call "MicroPulse - dof decoder.vi"("dof"=w1352) -> ("String"=w1351:string, "DOF"=w1328:T7)  [unwired: 3 in]
          n427 = call "MicroPulse - decode voltage sets.vi"("U8"=w1321) -> ("voltages"=w1347:string, "Voltages"=w1327:T11)  [unwired: 3 in]
          n428 = call "MicroPulse - decode IF card sets.vi"("U8"=w1321) -> ("card info"=w1320:string, "Interface Cards"=w1319:T8[])  [unwired: 3 in]
          n429 = Format Into String(format string="System Type: %s\nSerial Number: %d\nChannels PA/Conv:  %d/%d\nTx Buffer Size: %d MB\nDefault Sample Frequency: %dMHz\nActual Sample Frequency: %dMHz\nDefault DOF: %s\nActual DOF: %s\nSystem Error: %s\n\n-------------------\nSoftware Versions\n-------------------\n%s\n\n-----------------\nSystem Voltages\n-----------------\n%s\n\nSystem Temperature: %d °C\nProcessor Temperature: %d °C\nSlave SystemTemperature: %d °C\nSlave Processor Temperature: %d °C\n\n------------------------------\nSystem Interface Cards X%d\n------------------------------%s\nMessage Length: %dbytes", initial string="---------------------\nSystem Information\n---------------------\n", w1338, w1306, w1334, w1333, w1332, w1331, w1330, w1353, w1351, w1311, w1312, w1347, w1326, w1325, w1324, w1323, w1322, w1320, w1339) -> (resulting string=w1366:string)  [unwired: 1 in, 1 out]
          n430 = Bundle By Name(cluster=w1313, "System Type"=w1335, "Serial No."=w1306, "Channels.PA"=w1334, "Channels.Conv"=w1333, "Tx Buffer Size"=w1332, "Sample Frequency.Default"=w1331, "Sample Frequency.Actual"=w1330, "Data Output Format.Default"=w1329, "Data Output Format.Actual"=w1328, "System Error"=w1311, "Voltages"=w1327, "Temperatures.System"=w1326, "Temperatures.Processor"=w1325, "Temperatures.Slave Sys"=w1324, "Temperatures.Slave Proc"=w1323, "No. of Cards"=w1322, "Interface Cards"=w1319, "Software Versions"=w1312) -> (w1336:T5)
        }
      }
      n431 = Select(t=w842, s=w839, f="") -> (s? t:f=w841:string)
    }
    frame Default {
      w1380 = TRUE  # Warning
      # "Message header byte not recognised."
      n432 = Format Into String(format string="%02x", initial string="Message header byte not recognised: 0x", w1377) -> (resulting string=w1379:string)  [unwired: 1 in, 1 out]
      n433 = call <vilib>:"Error Cluster From Error Code.vi"("is warning? (False)"=w1380, "error message (\"\")"=w1379, "error code (0)"=7003 ("custom error code")) -> ("error out"=w1382:errorcluster)  [unwired: 6 in]
    }
  }
  "System Status" <- w1
  "reported msg length" <- w12
  "Axis Status" <- w16
  "Instrument Message" <- w7
  "message header" <- w3
  n434 = Bundle By Name(cluster=w9, "Message Header"=w3, "Error Message"=w2) -> (w4:T9)
  n435 = feedback-in #1(w1) -> ()
  n436 = feedback-in #2(w16) -> ()
  n437 = feedback-in #3(w4) -> ()
  n438 = call "MP - add Pos and MIP to encoder status.vi"("Axis Status"=w16, "scan data info"=w4) -> ("scan data info"=→"scan data info":T9)  [unwired: 9 in]
  n439 = Merge Errors(w6, "error in (no error)") -> (→"error out":errorcluster)
